vi "TorsionTester.vi"() -> ()   [LabVIEW 2020]
uses:
  C:/Users/elm2733/Box/Rausch Lab/LabView Files/Biaxial Device/MotorPlusLoadCells2 Folder v2016/FUTEK USB DLL.dll
  Box/Rausch Lab/LabView Files/Biaxial Device/MotorPlusLoadCells2 Folder v2016/FUTEK USB DLL.dll
  aec8d69f-4215-41ae-99f2-a40d43009400.vi
  f842f3ff-62f7-4fe2-ab09-e212065798b6.vi
  79f05c57-3d67-4982-bbb2-fea1714bb2cf.vi
  <vilib>/Array/Sort 2D Array - Pop Stack.vi
  <vilib>/Array/Sort 2D Array - Push Stack.vi
  aec8d69f-4215-41ae-99f2-a40d43009400.vi/269d4b3b-47f5-49e3-8884-44851e4dd9d5.vi
  aec8d69f-4215-41ae-99f2-a40d43009400.vi/6d99389c-673d-4efb-bf33-19b32bcf4cf8.vi
  f842f3ff-62f7-4fe2-ab09-e212065798b6.vi/269d4b3b-47f5-49e3-8884-44851e4dd9d5.vi
  f842f3ff-62f7-4fe2-ab09-e212065798b6.vi/6d99389c-673d-4efb-bf33-19b32bcf4cf8.vi
  79f05c57-3d67-4982-bbb2-fea1714bb2cf.vi/269d4b3b-47f5-49e3-8884-44851e4dd9d5.vi
  79f05c57-3d67-4982-bbb2-fea1714bb2cf.vi/6d99389c-673d-4efb-bf33-19b32bcf4cf8.vi
  <vilib>/Utility/file.llb/Write Delimited Spreadsheet (string).vi
  <vilib>/Utility/file.llb/Write Delimited Spreadsheet (DBL).vi
  <vilib>/express/express arith-compare/Formula/XNode/ExpressFormulaBlockNode.xnode
  Box/Rausch Lab/LabView Files/Biaxial Device/MotorPlusLoadCells2 Folder v2016/Zaber A Series/Zaber A Series.lvlib
panel:
  in  "Uniaxial Compression Test":bool
  in  "Uniaxial Tensile Test":bool
  in  "Compression (mm)":dbl format="%#_13g"
  in  "1 Step Test Button":bool
  in  "Cyclic Test Button":bool
  out "error out":errorcluster
  in  "Home Z Motor":bool
  in  "Cycles":i32
  in  "Step Size (mm)":dbl format="%#_13g"
  in  "Down":bool=TRUE
  in  "Up":bool=TRUE
  out "Z Motor Initialized":bool=TRUE
  in  "Motor Speed (mm/s)":dbl format="%#_13g"
  out "Force Sensor (lbs)":dbl format="%#_13g"
  in  "Zero Force Sensor":bool
  in  "Exit Loop":bool=TRUE
  out "Uniaxial Test":bool=TRUE
  out "Uniaxial Cycles":dbl format="%#_13g"
  out "Force/Time":dbl[](graph)
  out "Get_Decimal Point 3":string
  out "Get_Fullscale_Load 3":string
  out "Get_Fullscale_Value 3":string
  out "Get_Offset_Load 3":string
  out "Get_Offset_Value 3":string
  out "1/x 3":dbl format="%#_13g"
  out "Displacement/Time":sgl[](graph)
  in  "Displacement (mm)":dbl format="%#_13g"
  in  "Z Motor":refnum<k7>(container)
  out "Saved Position":dbl[](array[numeric])
  out "Position (Degrees)":dbl=6.0
  in  "Jog Graphs":bool
  out "On/Off":bool
  in  "Record Data":bool
  in  "Save Folder Path":path=path "C:/Users/kv8453/Desktop/LabVIEW_project_PB_tester/Output"
  in  "Sample Name":string="trial"
  out "1/x 2":dbl
  in  "Sampling Rate (Hz)":dbl
  out "Torque Sensor (in-oz)":dbl
  in  "Zero Torque Sensor":bool
  in  "Save Button":bool
  out "Torque/Time":dbl[](graph)
  out "Get_Decimal Point 2":string
  out "Get_Fullscale_Load 2":string
  out "Get_Fullscale_Value 2":string
  out "Get_Offset_Load 2":string
  out "Get_Offset_Value 2":string
  out "1/x":dbl
  in  "Angle (Degrees)":dbl=6.0
  in  "Move Distance (Deg)":dbl=6.0
  in  "Jog Size (Degrees)":dbl=6.0
  out "Angle/Time":dbl[](graph)
  in  "Home Button":bool
  in  "CW Button":bool
  in  "CCW Button":bool
  in  "Speed (Deg/s)":dbl=6.0
  out "Current Cycle":dbl
  in  "Cycles":i32=3
  in  "Quit":bool
  in  "VISA resource name":refnum<visa-resource-name>="COM4"
  # "Torsional Shear Tester                  X                       Uniaxial Tensile Tester"
  # "Rotation Stage = Yellow"
  # "Z Stage = Blue"
  # "Manuel Rausch"
  # "Ethan Maddin"
  # "Jog"
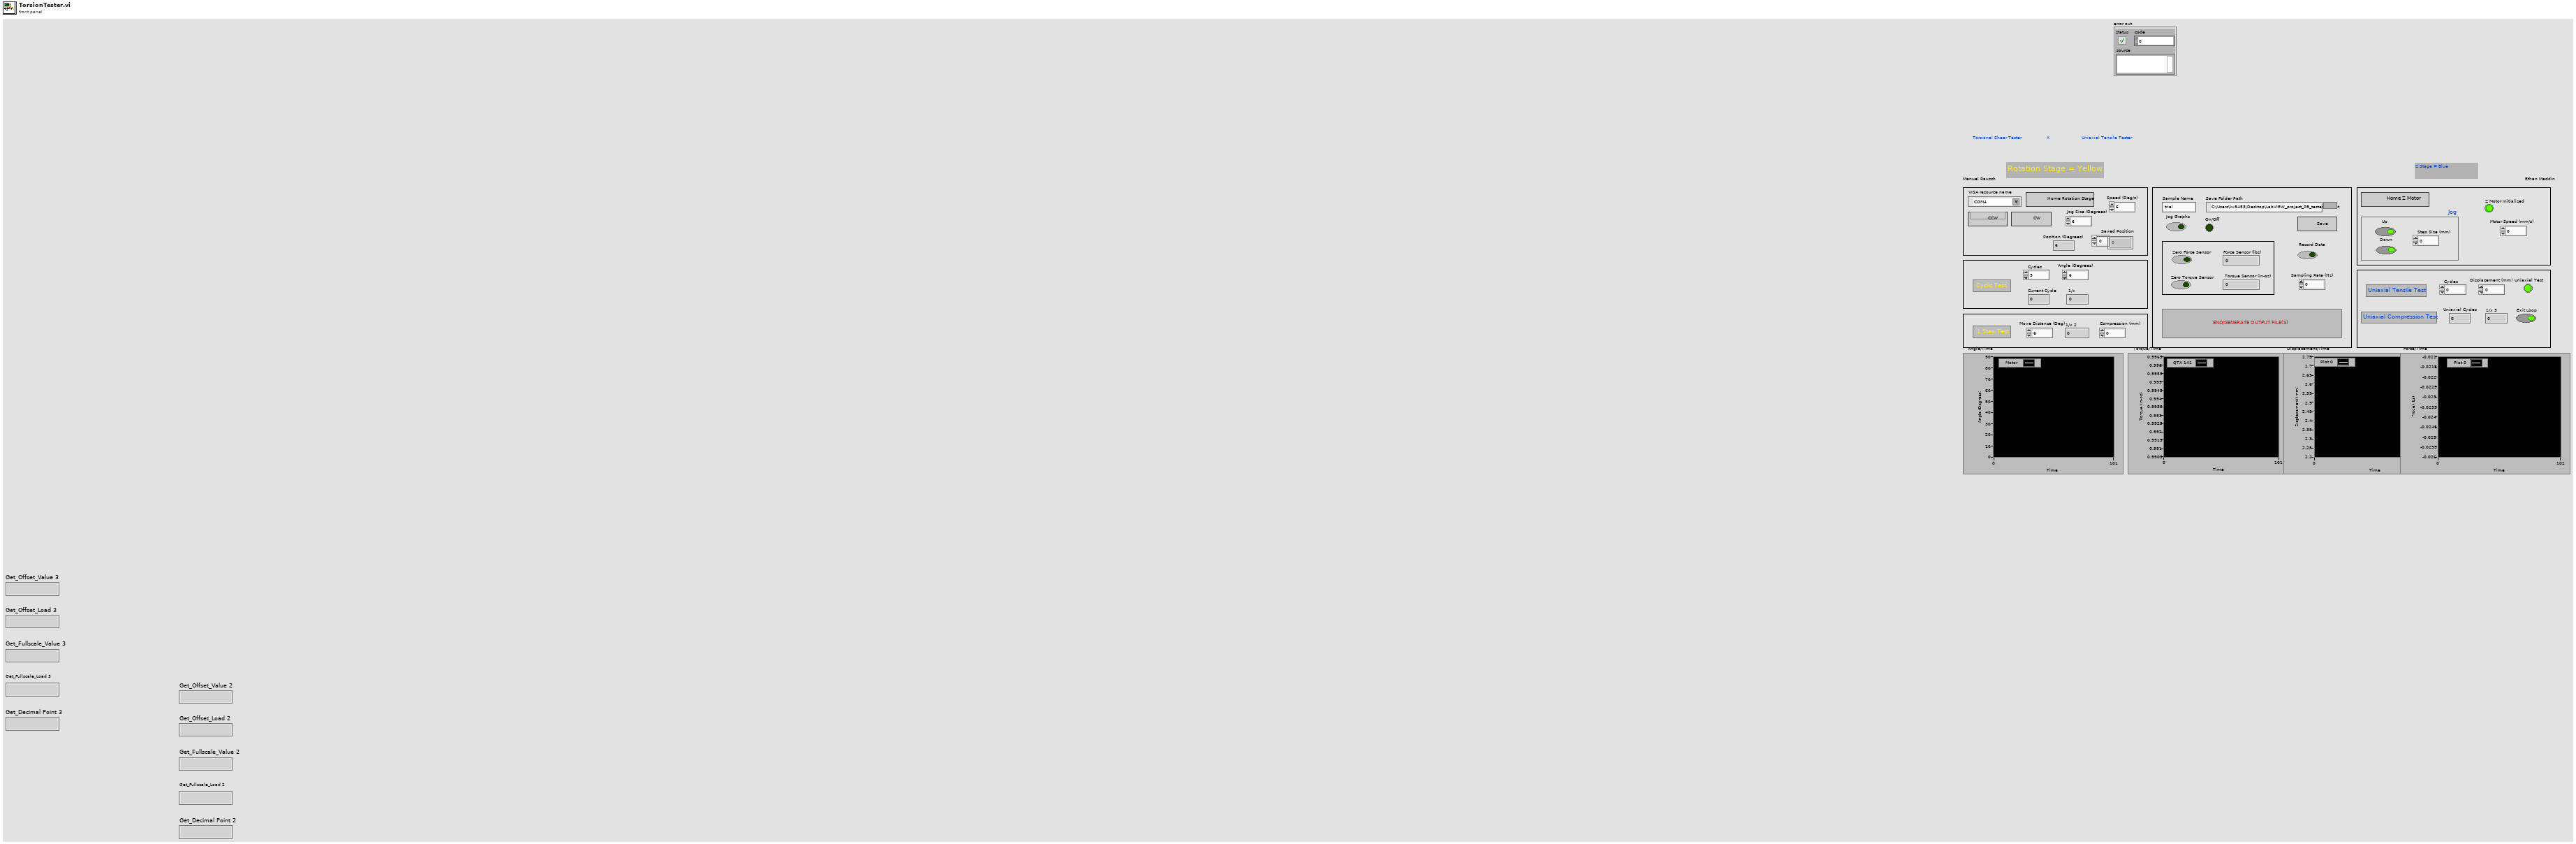
[diagram p1: front panel]
types:
  T1 = enum8{"Enabled", "Disabled", "Disabled and Grayed Out"}
  T2 = cluster{i32, i32, i32, i32, "new reference":refnum<k24>, "DeviceHandle":string, dbl}
  T3 = cluster{"new reference":refnum<k24>, "DeviceHandle":string}
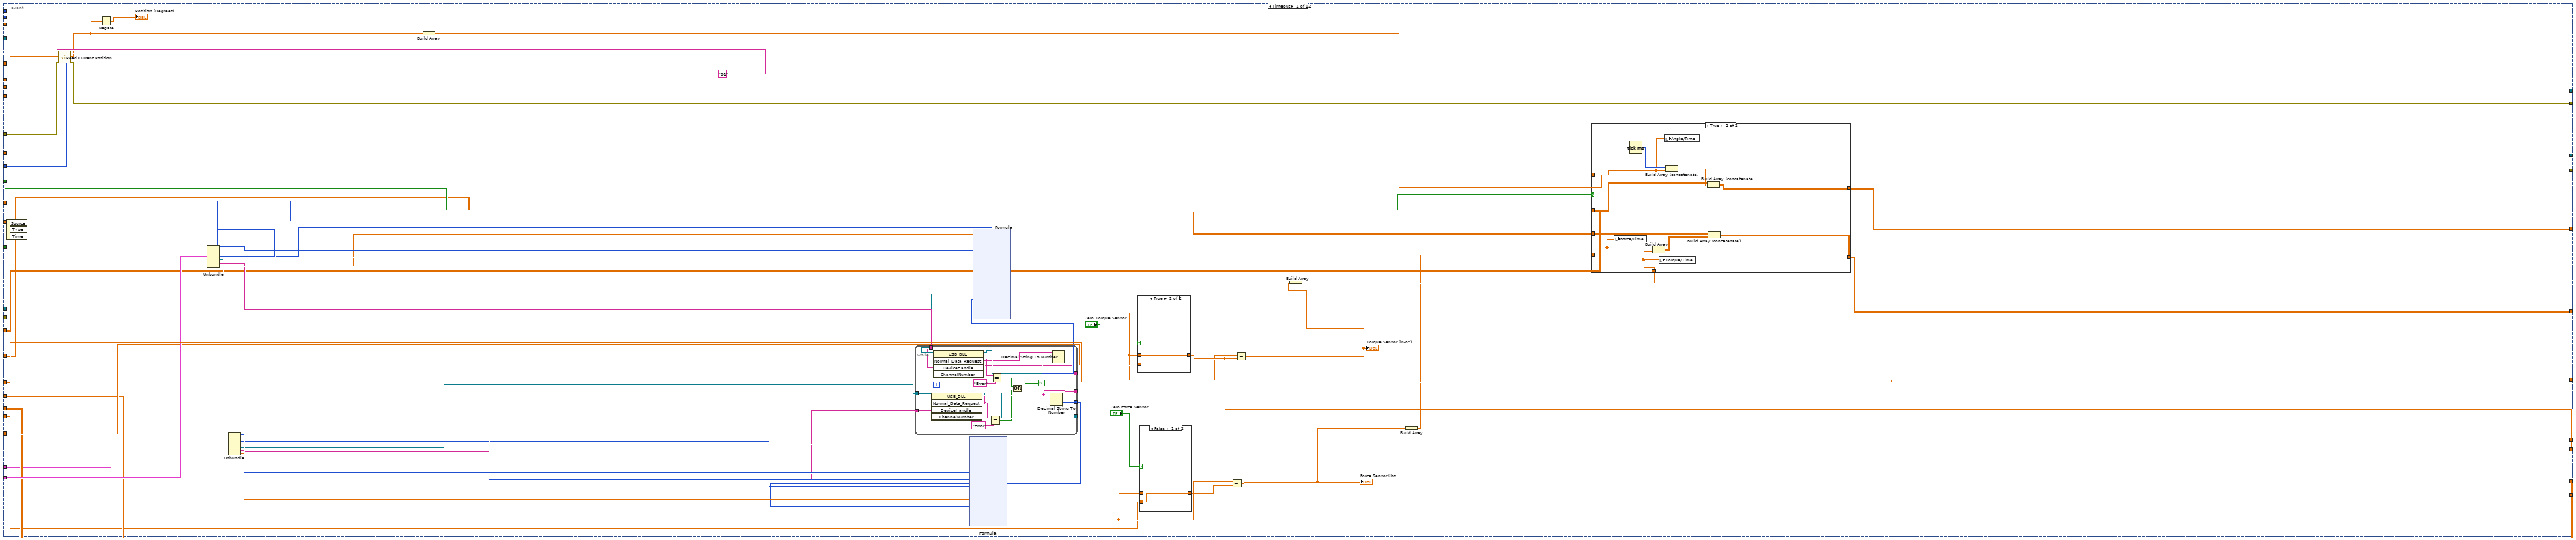
[diagram p2: hidden frame]
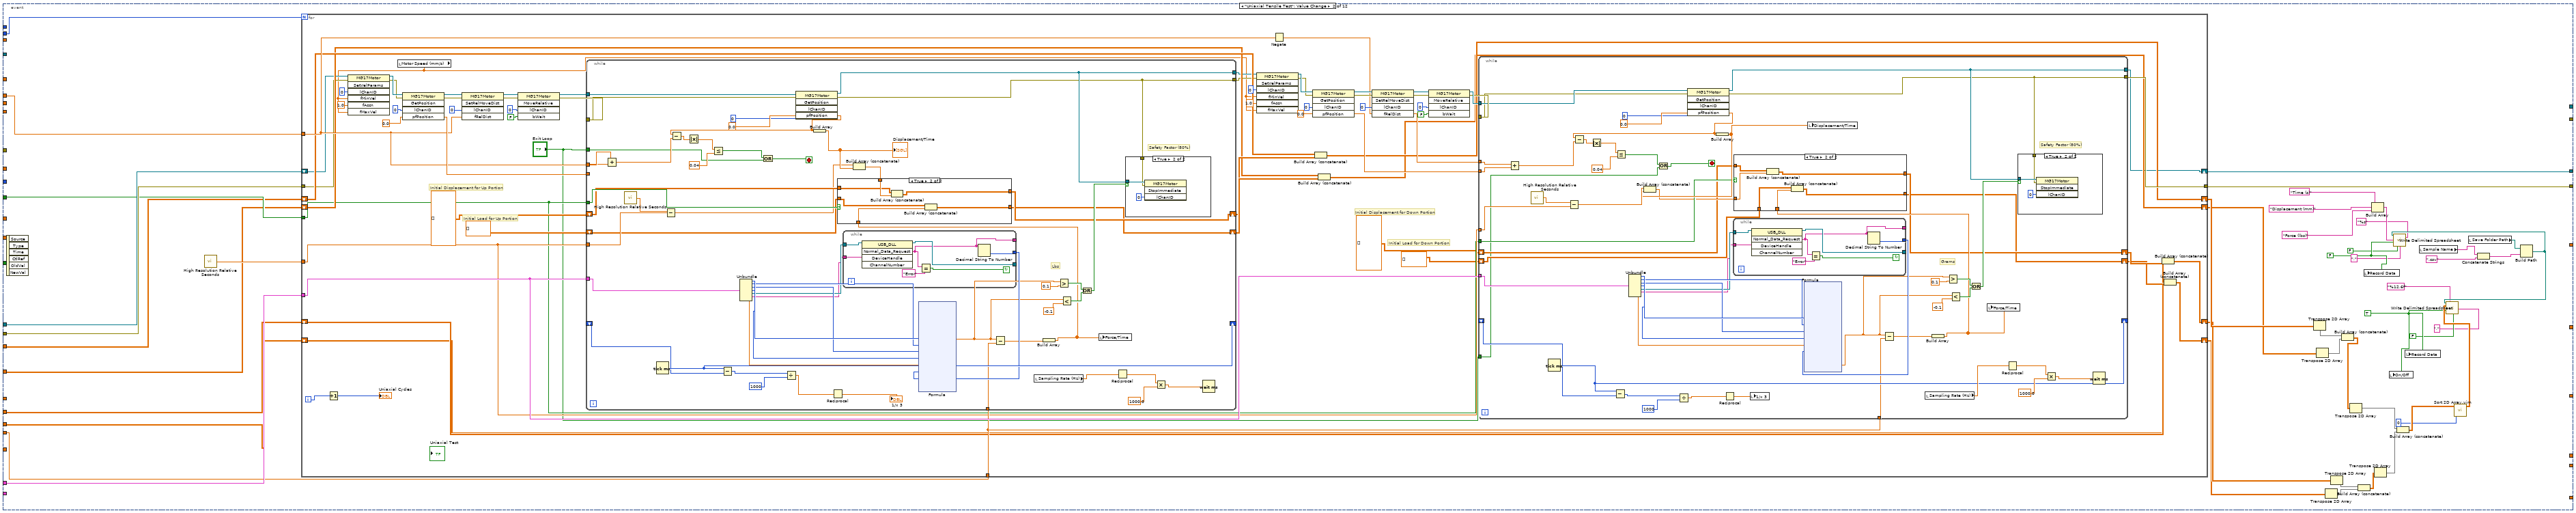
[diagram p6: hidden frame]
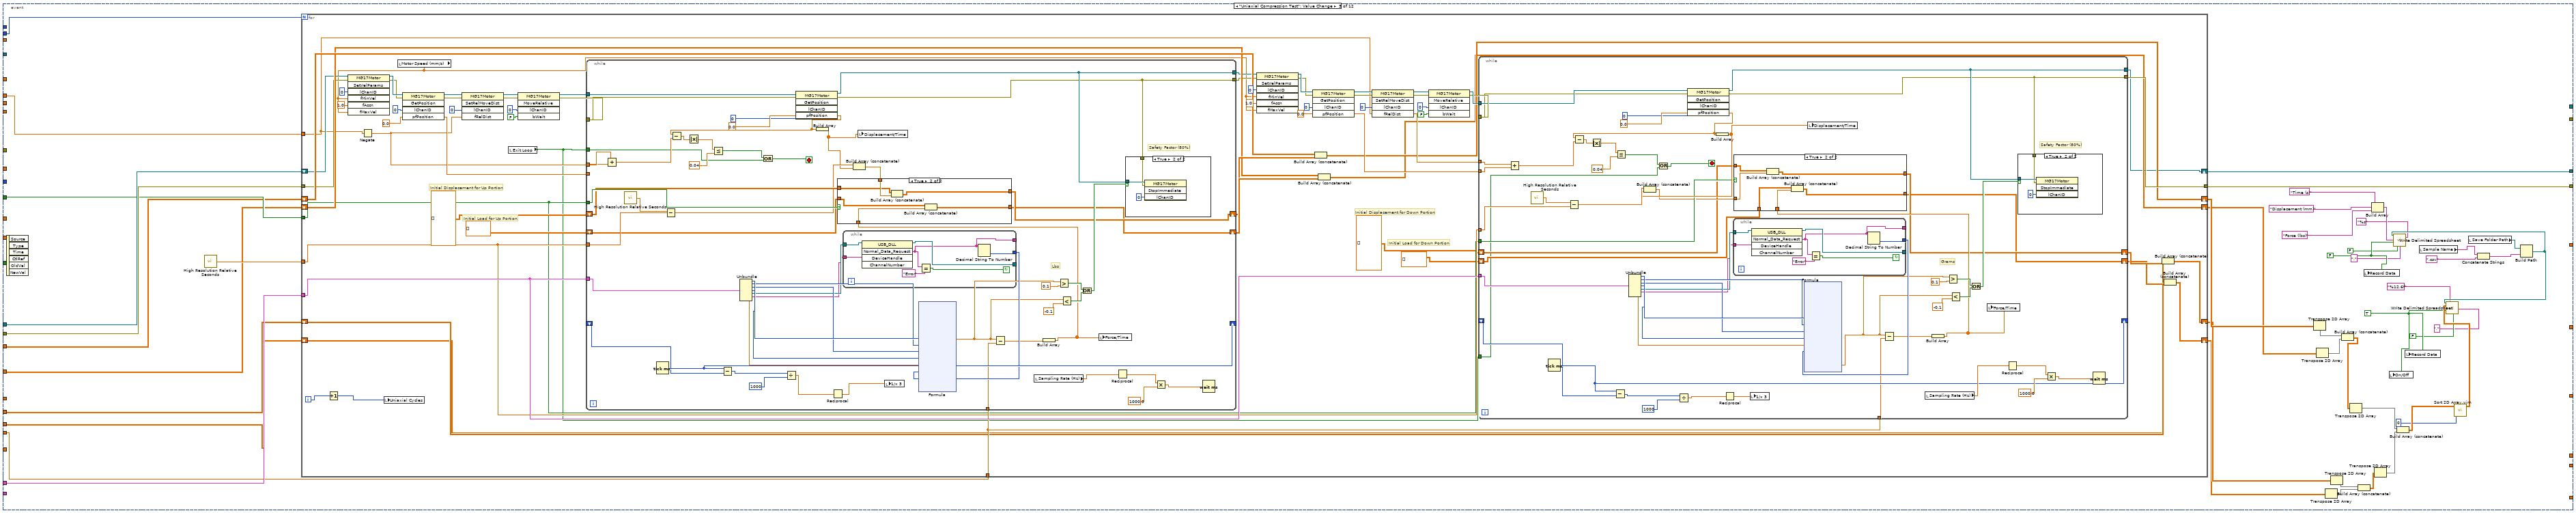
[diagram p11: hidden frame]
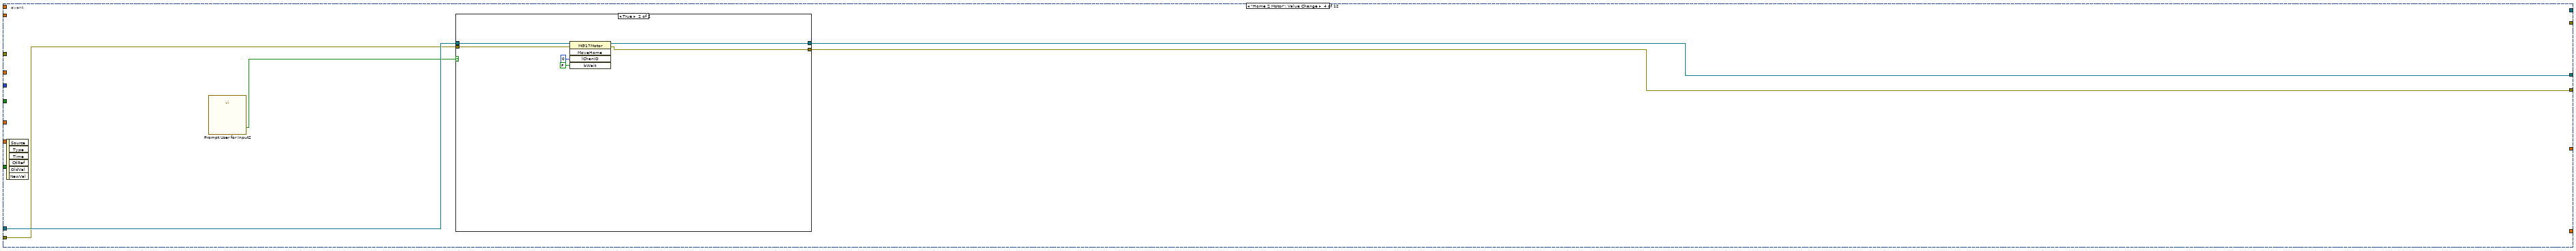
[diagram p16: hidden frame]
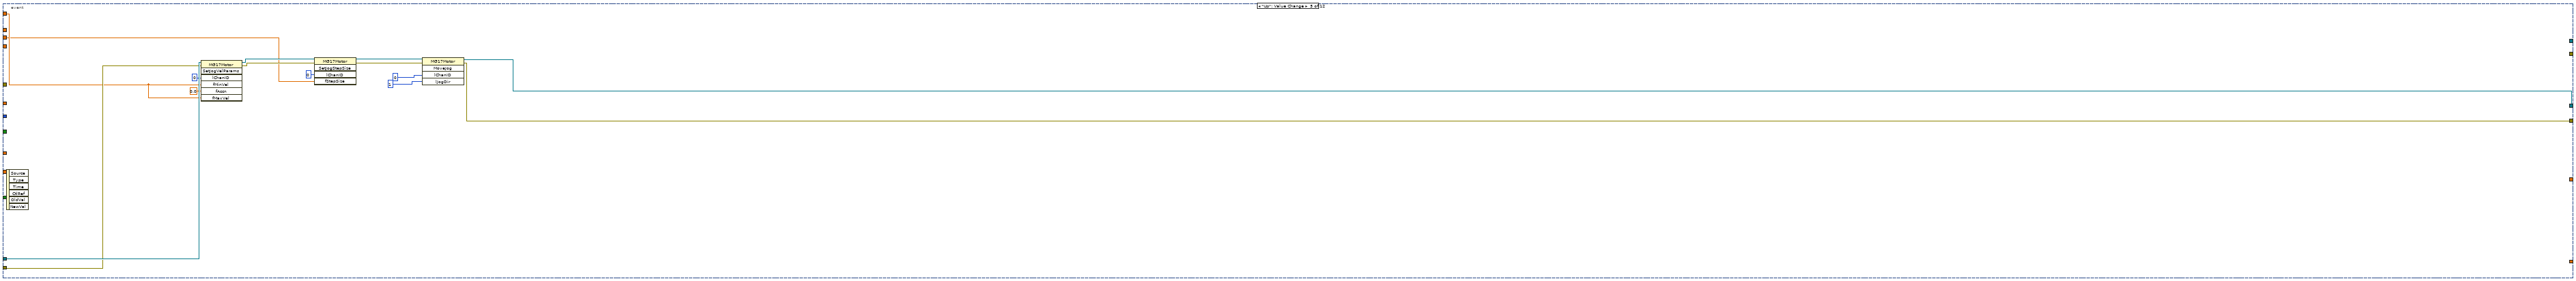
[diagram p18: hidden frame]
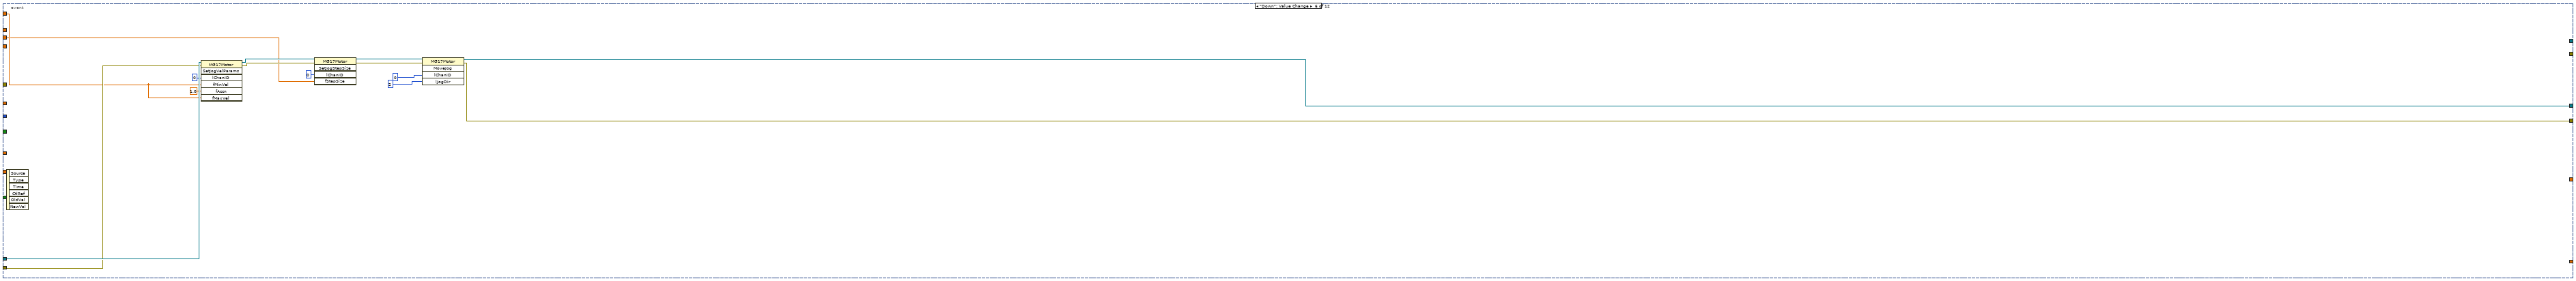
[diagram p19: hidden frame]
diagram:
  # "Sensor Data 2"
  # "Motor Exporting Data 2"
  # "Sensor Data 1"
  # "Motor Exporting Data 1"
  n1 = flat-sequence {
    tunnel: [w71] -> w22
    tunnel: [w70] -> w19
    tunnel: [dbl[] []] -> w21
    tunnel: [w51] -> w16
    tunnel: [w28] -> w7
    tunnel: [w27] -> w6
    tunnel: [w29] -> w4
    frame #0 {
      n2 = invoke on="Down" class="Bool (strict)" method="Reinit To Default"() -> ()  [unwired: 3 in, 3 out]
      n3 = invoke on="On/Off" class="Bool (strict)" method="Reinit To Default"() -> ()  [unwired: 3 in, 3 out]
      n4 = invoke on="Up" class="Bool (strict)" method="Reinit To Default"() -> ()  [unwired: 3 in, 3 out]
      n5 = invoke on="Uniaxial Test" class="Bool (strict)" method="Reinit To Default"() -> ()  [unwired: 3 in, 3 out]
      n6 = invoke on="Z Motor Initialized" class="Bool (strict)" method="Reinit To Default"() -> ()  [unwired: 3 in, 3 out]
    }
    frame #1 {
      n7 = constructor class="USB_DLL"() -> (reference out=w59:refnum<k24>)  [unwired: 3 in, 2 out]
      n8 = constructor class="USB_DLL"() -> (reference out=w37:refnum<k24>)  [unwired: 3 in, 2 out]
      n9 = invoke class="USB_DLL" method="Open_Device_Connection"(reference=w59, "SerialNumber"="1016700" ("Enter Serial Number")) -> (reference out=w61:refnum<k24>)  [unwired: 2 in, 3 out]
      n10 = invoke class="USB_DLL" method="Open_Device_Connection"(reference=w37, "SerialNumber"="905894" ("Enter Serial Number")) -> (reference out=w39:refnum<k24>)  [unwired: 2 in, 3 out]
      n11 = property class="USB_DLL"(reference=w61) -> (reference out=w67:refnum<k24>, "DeviceHandle"=w52:string)  [unwired: 1 in, 1 out]
      n12 = property class="USB_DLL"(reference=w39) -> (reference out=w45:refnum<k24>, "DeviceHandle"=w30:string)  [unwired: 1 in, 1 out]
      n13 = while {
        tunnel: w67 -> [w143]
        tunnel: w52 -> [w142]
        tunnel: [w138] -> w58
        tunnel: [w137] -> w65
        stop <- w139 continue-if-true
        # "Get_Offset_Value is used to read the ADC value stored in the USB device for a zero mV/V load."
        n14 = invoke class="USB_DLL" method="Get_Offset_Value"(reference=w143, "DeviceHandle"=w142) -> (reference out=w137:refnum<k24>, "Get_Offset_Value"=w141:string)  [unwired: 3 in, 3 out]
        "Get_Offset_Value 2" <- w141
        n15 = Equal?(x=w141, y="Error") -> (x = y?=w139:bool)
        n16 = Decimal String To Number(string=w141) -> (number=w138:i32)  [unwired: 2 in, 1 out]
      }
      n17 = while {
        tunnel: w45 -> [w108]
        tunnel: w30 -> [w107]
        tunnel: [w103] -> w36
        tunnel: [w102] -> w43
        stop <- w104 continue-if-true
        # "Get_Offset_Value is used to read the ADC value stored in the USB device for a zero mV/V load."
        n18 = invoke class="USB_DLL" method="Get_Offset_Value"(reference=w108, "DeviceHandle"=w107) -> (reference out=w102:refnum<k24>, "Get_Offset_Value"=w106:string)  [unwired: 3 in, 3 out]
        "Get_Offset_Value 3" <- w106
        n19 = Equal?(x=w106, y="Error") -> (x = y?=w104:bool)
        n20 = Decimal String To Number(string=w106) -> (number=w103:i32)  [unwired: 2 in, 1 out]
      }
      n21 = while {
        tunnel: [w133] -> w57
        tunnel: [w132] -> w64
        tunnel: w65 -> [w131]
        tunnel: w52 -> [w130]
        stop <- w134 continue-if-true
        # "Get_Offset_Load is used to read the capacity of the zero load value stored in the USB device."
        n22 = invoke class="USB_DLL" method="Get_Offset_Load"(reference=w131, "DeviceHandle"=w130) -> (reference out=w132:refnum<k24>, "Get_Offset_Load"=w136:string)  [unwired: 3 in, 3 out]
        "Get_Offset_Load 2" <- w136
        n23 = Equal?(x=w136, y="Error") -> (x = y?=w134:bool)
        n24 = Decimal String To Number(string=w136) -> (number=w133:i32)  [unwired: 2 in, 1 out]
      }
      n25 = while {
        tunnel: [w98] -> w35
        tunnel: [w97] -> w42
        tunnel: w43 -> [w96]
        tunnel: w30 -> [w95]
        stop <- w99 continue-if-true
        # "Get_Offset_Load is used to read the capacity of the zero load value stored in the USB device."
        n26 = invoke class="USB_DLL" method="Get_Offset_Load"(reference=w96, "DeviceHandle"=w95) -> (reference out=w97:refnum<k24>, "Get_Offset_Load"=w101:string)  [unwired: 3 in, 3 out]
        "Get_Offset_Load 3" <- w101
        n27 = Equal?(x=w101, y="Error") -> (x = y?=w99:bool)
        n28 = Decimal String To Number(string=w101) -> (number=w98:i32)  [unwired: 2 in, 1 out]
      }
      n29 = while {
        tunnel: [w126] -> w56
        tunnel: [w125] -> w63
        tunnel: w64 -> [w124]
        tunnel: w52 -> [w123]
        stop <- w127 continue-if-true
        # "Get_Fullscale_Value is used to read the ADC value stored in the USB device for a full load."
        n30 = invoke class="USB_DLL" method="Get_Fullscale_Value"(reference=w124, "DeviceHandle"=w123) -> (reference out=w125:refnum<k24>, "Get_Fullscale_Value"=w129:string)  [unwired: 3 in, 3 out]
        "Get_Fullscale_Value 2" <- w129
        n31 = Equal?(x=w129, y="Error") -> (x = y?=w127:bool)
        n32 = Decimal String To Number(string=w129) -> (number=w126:i32)  [unwired: 2 in, 1 out]
      }
      n33 = while {
        tunnel: [w91] -> w34
        tunnel: [w90] -> w41
        tunnel: w42 -> [w89]
        tunnel: w30 -> [w88]
        stop <- w92 continue-if-true
        # "Get_Fullscale_Value is used to read the ADC value stored in the USB device for a full load."
        n34 = invoke class="USB_DLL" method="Get_Fullscale_Value"(reference=w89, "DeviceHandle"=w88) -> (reference out=w90:refnum<k24>, "Get_Fullscale_Value"=w94:string)  [unwired: 3 in, 3 out]
        "Get_Fullscale_Value 3" <- w94
        n35 = Equal?(x=w94, y="Error") -> (x = y?=w92:bool)
        n36 = Decimal String To Number(string=w94) -> (number=w91:i32)  [unwired: 2 in, 1 out]
      }
      n37 = property class="MG17Motor"(reference="Z Motor", error in=errorcluster {"status"=FALSE, "code"=0, "source"=""}, "HWSerialNum"=27262533 ("HWSerialNum 3")) -> (reference out=w24:refnum<k7>, error out=w23:errorcluster)
      n38 = invoke class="MG17Motor" method="StartCtrl"(reference=w24, error in=w23) -> (reference out=w46:refnum<k7>, error out=w47:errorcluster)  [unwired: 1 in, 1 out]
      n39 = while {
        tunnel: [w119] -> w55
        tunnel: [w118] -> w62
        tunnel: w63 -> [w117]
        tunnel: w52 -> [w116]
        stop <- w120 continue-if-true
        # "Get_Fullsacle_Load is used to read the capacity of the full load value stored in the USB device."
        n40 = invoke class="USB_DLL" method="Get_Fullscale_Load"(reference=w117, "DeviceHandle"=w116) -> (reference out=w118:refnum<k24>, "Get_Fullscale_Load"=w122:string)  [unwired: 3 in, 3 out]
        "Get_Fullscale_Load 2" <- w122
        n41 = Equal?(x=w122, y="Error") -> (x = y?=w120:bool)
        n42 = Decimal String To Number(string=w122) -> (number=w119:i32)  [unwired: 2 in, 1 out]
      }
      n43 = while {
        tunnel: [w84] -> w33
        tunnel: [w83] -> w40
        tunnel: w41 -> [w82]
        tunnel: w30 -> [w81]
        stop <- w85 continue-if-true
        # "Get_Fullsacle_Load is used to read the capacity of the full load value stored in the USB device."
        n44 = invoke class="USB_DLL" method="Get_Fullscale_Load"(reference=w82, "DeviceHandle"=w81) -> (reference out=w83:refnum<k24>, "Get_Fullscale_Load"=w87:string)  [unwired: 3 in, 3 out]
        "Get_Fullscale_Load 3" <- w87
        n45 = Equal?(x=w87, y="Error") -> (x = y?=w85:bool)
        n46 = Decimal String To Number(string=w87) -> (number=w84:i32)  [unwired: 2 in, 1 out]
      }
      n47 = invoke class="MG17Motor" method="GetHWCommsOK"(reference=w46, error in=w47, "pbCommsOK"=FALSE) -> (reference out=w28:refnum<k7>, error out=w27:errorcluster, "pbCommsOK"=→"Z Motor Initialized":bool)  [unwired: 1 in, 1 out]
      n48 = call "Initialize.vi"("error in (no error)"=errorcluster {"status"=FALSE, "code"=0, "source"=""}, "VISA resource name"="VISA resource name") -> ("error out"=w70:errorcluster, "VISA resource name out"=w71:refnum<visa-resource-name>)  [unwired: 8 in]
      n49 = while {
        tunnel: [w112] -> w66
        tunnel: [w111] -> w53
        tunnel: w62 -> [w110]
        tunnel: w52 -> [w109]
        stop <- w113 continue-if-true
        # "Get_Decimal_Point is used to read the position of the decimal point stored in the USB device.  The decimal point is then turned into a negative power of 10."
        n50 = invoke class="USB_DLL" method="Get_Decimal_Point"(reference=w110, "DeviceHandle"=w109) -> (reference out=w111:refnum<k24>, "Get_Decimal_Point"=w115:string)  [unwired: 3 in, 3 out]
        "Get_Decimal Point 2" <- w115
        n51 = Equal?(x=w115, y="Error") -> (x = y?=w113:bool)
        n52 = Decimal String To Number(string=w115) -> (number=w112:i32)  [unwired: 2 in, 1 out]
      }
      n53 = while {
        tunnel: [w77] -> w44
        tunnel: [w76] -> w31
        tunnel: w40 -> [w75]
        tunnel: w30 -> [w74]
        stop <- w78 continue-if-true
        # "Get_Decimal_Point is used to read the position of the decimal point stored in the USB device.  The decimal point is then turned into a negative power of 10."
        n54 = invoke class="USB_DLL" method="Get_Decimal_Point"(reference=w75, "DeviceHandle"=w74) -> (reference out=w76:refnum<k24>, "Get_Decimal_Point"=w80:string)  [unwired: 3 in, 3 out]
        "Get_Decimal Point 3" <- w80
        n55 = Equal?(x=w80, y="Error") -> (x = y?=w78:bool)
        n56 = Decimal String To Number(string=w80) -> (number=w77:i32)  [unwired: 2 in, 1 out]
      }
      n57 = Power Of 10(x=w66) -> (10^x=w54:dbl)
      n58 = Power Of 10(x=w44) -> (10^x=w32:dbl)
      n59 = property on="Home Button" class="Bool"("DisabledEnum"=T1."Enabled" ("Disabled")) -> ()  [unwired: 2 in, 2 out]
      n60 = Bundle(w58, w57, w56, w55, "new reference"=w53, "DeviceHandle"=w52, w54) -> (w51:T2)  [unwired: 1 in]
      n61 = Bundle(w36, w35, w34, w33, "new reference"=w31, "DeviceHandle"=w30, w32) -> (w29:T2)  [unwired: 1 in]
    }
  }
  n62 = while {
    tunnel: w22 -> [w187]
    tunnel: [w184] -> w20
    shift-right: [w183] -> w13
    shift-left: w19 -> [w182]
    shift-right: [w164] -> w8
    shift-left: w21 -> [w181]
    shift-right: [w175] -> _
    shift-left: 0.0 -> [w177]
    shift-right: [w174] -> _
    shift-left: 0.0 -> [w176]
    tunnel: w16 -> [w173]
    tunnel: [w169] -> w15
    tunnel: [w168] -> w14
    tunnel: dbl[][] [] ("Array") -> [w163]
    tunnel: dbl[][] [] ("Array") -> [w161]
    tunnel: dbl[][] [] ("Array") -> [w160]
    tunnel: dbl[][] [] ("Array") -> [w159]
    tunnel: w6 -> [w156]
    tunnel: [w155] -> w5
    tunnel: w4 -> [w154]
    tunnel: [w150] -> w3
    tunnel: [w149] -> w2
    tunnel: w7 -> [w157]
    tunnel: [w147] -> w1
    stop <- "Quit" stop-if-true
    w185 = u16 4 items=["microsteps", "microns", "millimeters", "inches", "degrees"] ("Units (0: microsteps)")
    # "Uniaxial"
    # "Torsional Shear"
    n63 = Unbundle By Name(w173) -> ("new reference"=w172:refnum<k24>, "DeviceHandle"=w171:string)
    n64 = Unbundle By Name(w154) -> ("new reference"=w153:refnum<k24>, "DeviceHandle"=w152:string)
    n65 = event shown="[6] \"1 Step Test Button\": Value Change" {
      selector: _ -> [_ _ _ _ _ _ _ _ _ _ _ _]
      dyn-events: _ -> [_ _ _ _ _ _ _ _ _ _ _ _]
      timeout: u32 10 ("millisecond timer value") -> [_ _ _ _ _ _ _ _ _ _ _ _]
      tunnel: "Cycles" -> [_ _ _ _ _ _ _ w1249 _ _ _ _]
      tunnel: w187 -> [w234 _ _ _ _ _ w974 w1248 w1593 w1666 w1727 w1752]
      tunnel: 0.000234375 -> [w237 _ _ _ _ _ w972 w1247 w1596 w1667 _ w1754]
      tunnel: w185 -> [w236 _ _ _ _ _ w982 w1246 w1595 w1668 _ w1753]
      tunnel: [w232 _ _ _ _ _ w979 w1245 w1581 w1652 w1725 w1749] -> w184
      tunnel: [w231 _ _ _ _ _ w978 w1244 w1580 w1651 w1724 w1748] -> w183
      tunnel: w182 -> [w235 _ _ _ _ _ w973 w1243 w1592 w1665 w1728 w1751]
      tunnel: "Jog Size (Degrees)" -> [_ _ _ _ _ _ _ _ w1597 w1670 _ _]
      tunnel: w181 -> [w230 _ _ _ _ _ w960 w1242 w1590 w1662 w1735 _]
      tunnel: [w230 _ _ _ _ _ w959 w1242 w1590 w1662 w1735 w1745] -> w164
      tunnel: "Move Distance (Deg)" -> [_ _ _ _ _ _ w962 _ _ _ _ _]
      tunnel: "Angle (Degrees)" -> [_ _ _ _ _ _ _ w1241 _ _ _ _]
      tunnel: w177 -> [w192 w345 w636 _ _ _ w977 w1238 w1589 w1661 w1734 w1747]
      tunnel: w176 -> [w221 _ _ _ _ _ w976 w1237 w1588 w1660 w1733 w1746]
      tunnel: [_ _ _ _ _ _ w977 w1238 w1589 w1661 w1734 w1747] -> w175
      tunnel: [w220 _ _ _ _ _ w976 w1237 w1588 w1660 w1733 w1746] -> w174
      tunnel: w173 -> [w229 _ _ _ _ _ w975 w1239 w1584 w1655 _ _]
      tunnel: "Record Data" -> [_ w344 w635 _ _ _ w971 w1236 _ _ _ _]
      tunnel: [w216 _ _ _ _ _ _ _ w1587 w1659 w1732 _] -> _
      tunnel: w163 -> [w217 w342 w633 _ _ _ w968 w1235 w1587 w1659 w1732 _]
      tunnel: "Jog Graphs" -> [w215 _ _ _ _ _ _ _ _ _ _ _]
      tunnel: w161 -> [w213 w341 w632 _ _ _ w965 w1234 _ w1658 w1731 _]
      tunnel: [w212 _ _ _ _ _ _ _ _ w1658 w1731 _] -> _
      tunnel: w160 -> [w210 w340 w631 _ _ _ w964 w1233 w1586 w1657 w1730 _]
      tunnel: w159 -> [w209 w339 w630 _ _ _ w963 w1232 w1585 w1656 w1729 _]
      tunnel: [w210 _ _ _ _ _ w964 _ w1586 w1657 w1730 _] -> _
      tunnel: [w209 _ _ _ _ _ w963 _ w1585 w1656 w1729 _] -> _
      tunnel: "Displacement (mm)" -> [_ w348 w639 _ _ _ _ _ _ _ _ _]
      tunnel: w157 -> [_ w350 w641 w891 w914 w929 w954 _ _ _ _ _]
      tunnel: w156 -> [_ w349 w640 w890 w913 w928 w953 _ _ _ _ _]
      tunnel: [_ w306 w597 w888 w901 w916 w945 _ _ _ _ _] -> w147
      tunnel: [_ w347 w638 w887 w900 w915 w944 _ _ _ _ _] -> w155
      tunnel: w154 -> [w205 w346 w637 _ _ _ w956 w1198 _ _ _ _]
      tunnel: "Motor Speed (mm/s)" -> [_ _ _ _ w910 w925 w952 _ _ _ _ _]
      tunnel: "Step Size (mm)" -> [_ _ _ _ w906 w921 _ _ _ _ _ _]
      tunnel: "Cycles" -> [_ w305 w596 _ _ _ _ _ _ _ _ _]
      tunnel: "Compression (mm)" -> [_ _ _ _ _ _ w955 _ _ _ _ _]
      event Timeout {
        n66 = event-data() -> ()  [unwired: 1 in, 3 out]
        n67 = call "Read Current Position.vi"("Units (0: microsteps)"=w236, "error in (no error)"=w235, "Device and Axis"="01", "Microstep Size (0)"=w237, "VISA resource name"=w234) -> ("error out"=w231:errorcluster, "Position"=w208:dbl, "VISA resource name out"=w232:refnum<visa-resource-name>)  [unwired: 4 in]
        n68 = Negate(x=w208) -> (-x=→"Position (Degrees)":dbl)
        n69 = Unbundle(w229) -> (w228:i32, w227:i32, w226:i32, w225:i32, "new reference"=w222:refnum<k24>, "DeviceHandle"=w223:string, w224:dbl)
        n70 = Unbundle(w205) -> (w203:i32, w202:i32, w201:i32, w200:i32, "new reference"=w198:refnum<k24>, "DeviceHandle"=w197:string, w199:dbl)
        n71 = Build Array(w208) -> (w218:dbl[])
        n72 = while {
          tunnel: [w285] -> w219
          tunnel: w222 -> [w284]
          tunnel: [w283] -> _
          tunnel: w223 -> [w282]
          tunnel: [w281] -> _
          tunnel: w198 -> [w279]
          tunnel: w197 -> [w278]
          tunnel: [w277] -> _
          tunnel: [w276] -> _
          tunnel: [w275] -> w196
          stop <- w272 continue-if-true
          n73 = invoke class="USB_DLL" method="Normal_Data_Request"(reference=w279, "DeviceHandle"=w278) -> (reference out=w277:refnum<k24>, "Normal_Data_Request"=w276:string)  [unwired: 3 in, 3 out]
          n74 = invoke class="USB_DLL" method="Normal_Data_Request"(reference=w284, "DeviceHandle"=w282) -> (reference out=w283:refnum<k24>, "Normal_Data_Request"=w281:string)  [unwired: 3 in, 3 out]
          n75 = Equal?(x=w276, y="Error") -> (x = y?=w273:bool)
          n76 = Equal?(x=w281, y="Error") -> (x = y?=w274:bool)
          n77 = Or(x=w274, y=w273) -> (x .or. y?=w272:bool)
          n78 = Decimal String To Number(string=w276) -> (number=w275:i32)  [unwired: 2 in, 1 out]
          n79 = Decimal String To Number(string=w281) -> (number=w285:i32)  [unwired: 2 in, 1 out]
        }
        n80 = xnode "Formula"("Get_Offset_Value"=w203, "Get_Offset_Load"=w202, "Get_Fullscale_Value"=w201, "Get_Fullscale_Load"=w200, "Get_Decimal_Point"=w199, "Normal_Data_Request"=w196) -> ("Result"=w194:dbl)  [unwired: 1 in, 1 out]
        n81 = xnode "Formula"("Get_Offset_Value"=w228, "Get_Offset_Load"=w227, "Get_Fullscale_Value"=w226, "Get_Fullscale_Load"=w225, "Get_Decimal_Point"=w224, "Normal_Data_Request"=w219) -> ("Result"=w214:dbl)  [unwired: 1 in, 1 out]
        n82 = case shown="True" "Zero Torque Sensor" {
          tunnel: w214 -> [_ w271]
          tunnel: [w270 w271] -> w220
          tunnel: w221 -> [w270 _]
          frame False {
          }
          frame True {
          }
        }
        n83 = case shown="False" "Zero Force Sensor" {
          tunnel: w194 -> [_ w239]
          tunnel: [w238 w239] -> w193
          tunnel: w192 -> [w238 _]
          frame False {
          }
          frame True {
          }
        }
        n84 = Subtract(x=w194, y=w193) -> (x-y=w191:dbl)
        "Force Sensor (lbs)" <- w191
        n85 = Subtract(x=w214, y=w220) -> (x-y=w204:dbl)
        "Torque Sensor (in-oz)" <- w204
        n86 = Build Array(w204) -> (w206:dbl[])
        n87 = Build Array(w191) -> (w190:dbl[])
        n88 = case shown="True" w215 {
          tunnel: w218 -> [_ w265]
          tunnel: w217 -> [w259 w266]
          tunnel: [w259 w268] -> w216
          tunnel: w206 -> [_ w261]
          tunnel: w213 -> [w258 w263]
          tunnel: [w258 w262] -> w212
          tunnel: w190 -> [_ w260]
          frame False {
          }
          frame True {
            n89 = local write "Force/Time"(w260) -> ()
            n90 = Tick Count (ms)() -> (millisecond timer value=w269:u32)
            n91 = Build Array(w260, w261) -> (w264:dbl[][])
            n92 = local write "Torque/Time"(w261) -> ()
            n93 = local write "Angle/Time"(w265) -> ()
            n94 = Build Array (concatenate)(w269, w265) -> (w267:dbl[])
            n95 = Build Array (concatenate)(w266, w267) -> (w268:dbl[][])
            n96 = Build Array (concatenate)(w263, w264) -> (w262:dbl[][])
          }
        }
      }
      event "Uniaxial Tensile Test": Value Change {
        w325 = FALSE
        w319 = TRUE ("append to file? (new file:F)")
        n97 = event-data() -> ()  [unwired: 1 in, 6 out]
        n98 = call <vilib>:"High Resolution Relative Seconds.vi"() -> ("relative seconds"=w343:dbl)
        n99 = for {
          N: w305 -> [_]
          tunnel: w348 -> [w396]
          tunnel: w346 -> [w393]
          tunnel: w345 -> [w388]
          tunnel: w349 -> [w362]
          tunnel: [w387] -> w347
          tunnel: w344 -> [w376]
          tunnel: w343 -> [w385]
          shift-right: [w378] -> w313
          shift-left: w342 -> [w380]
          shift-right: [w377] -> w312
          shift-left: w341 -> [w379]
          shift-right: [w369] -> w311
          shift-left: w340 -> [w371]
          shift-right: [w368] -> w310
          shift-left: w339 -> [w370]
          shift-right: [w352] -> w306
          shift-left: w350 -> [w363]
          i -> [w406]
          # "Initial Displacement for Down Portion"
          # "Initial Load for Down Portion"
          # "Initial Displacement for Up Portion"
          # "Initial Load for Up Portion"
          n100 = Increment(x=w406) -> (x+1=→"Uniaxial Cycles":i32)
          n101 = local read "Motor Speed (mm/s)"() -> (w353:dbl)
          n102 = invoke class="MG17Motor" method="SetVelParams"(reference=w363, error in=w362, "lChanID"=0, "fMinVel"=w353, "fAccn"=sgl 1.0, "fMaxVel"=w353) -> (reference out=w361:refnum<k7>, error out=w360:errorcluster)  [unwired: 1 in, 5 out]
          n103 = invoke class="MG17Motor" method="GetPosition"(reference=w361, error in=w360, "lChanID"=0, "pfPosition"=sgl 0.0) -> (reference out=w410:refnum<k7>, error out=w409:errorcluster, "pfPosition"=w405:sgl)  [unwired: 1 in, 2 out]
          n104 = invoke class="MG17Motor" method="SetRelMoveDist"(reference=w410, error in=w409, "lChanID"=0, "fRelDist"=w396) -> (reference out=w414:refnum<k7>, error out=w413:errorcluster)  [unwired: 1 in, 3 out]
          n105 = invoke class="MG17Motor" method="MoveRelative"(reference=w414, error in=w413, "lChanID"=0, "bWait"=FALSE) -> (reference out=w351:refnum<k7>, error out=w407:errorcluster)  [unwired: 1 in, 3 out]
          n106 = while {
            tunnel: w407 -> [w559]
            shift-right: [w548] -> _
            shift-left: _ -> [w547]
            tunnel: [w523] -> w359
            tunnel: [w521] -> w358
            tunnel: w393 -> [w546]
            tunnel: w388 -> [w537]
            tunnel: w396 -> [w535]
            tunnel: w405 -> [w534]
            tunnel: w385 -> [w519]
            tunnel: w376 -> [w518]
            shift-right: [w511] -> w381
            shift-left: dbl[][] [] ("Array") -> [w517]
            shift-right: [w510] -> w382
            shift-left: dbl[][] [] ("Array") -> [w516]
            tunnel: "Exit Loop" -> [w507]
            tunnel: w351 -> [w506]
            stop <- w508 stop-if-true
            # "Safety Factor (80%)"
            # "Lbs"
            n107 = Add(x=w535, y=w534) -> (x+y=w532:dbl)
            n108 = call <vilib>:"High Resolution Relative Seconds.vi"() -> ("relative seconds"=w520:dbl)
            n109 = Tick Count (ms)() -> (millisecond timer value=w548:u32)
            n110 = Subtract(x=w520, y=w519) -> (x-y=w514:dbl)
            n111 = Subtract(x=w548, y=w547) -> (x-y=w552:u32)
            n112 = Unbundle(w546) -> (w545:i32, w544:i32, w543:i32, w542:i32, "new reference"=w540:refnum<k24>, "DeviceHandle"=w539:string, w541:dbl)
            n113 = Divide(x=w552, y=1000) -> (x/y=w550:dbl)
            n114 = invoke class="MG17Motor" method="GetPosition"(reference=w506, error in=w559, "lChanID"=0, "pfPosition"=sgl 0.0) -> (reference out=w523:refnum<k7>, error out=w521:errorcluster, "pfPosition"=w533:sgl)  [unwired: 1 in, 2 out]
            n115 = Subtract(x=w533, y=w532) -> (x-y=w530:dbl)
            n116 = Absolute Value(x=w530) -> (abs(x)=w529:dbl)
            n117 = Less Or Equal?(x=w529, y=0.04) -> (x <= y?=w509:bool)
            n118 = Or(x=w509, y=w507) -> (x .or. y?=w508:bool)
            n119 = Build Array(w533) -> (w515:sgl[])
            "Displacement/Time" <- w515
            n120 = Reciprocal(x=w550) -> (1/x=→"1/x 3":dbl)
            n121 = while {
              tunnel: [w594] -> _
              tunnel: [w593] -> _
              tunnel: [w592] -> w538
              tunnel: w539 -> [w591]
              tunnel: w540 -> [w590]
              stop <- w589 continue-if-true
              n122 = invoke class="USB_DLL" method="Normal_Data_Request"(reference=w590, "DeviceHandle"=w591) -> (reference out=w594:refnum<k24>, "Normal_Data_Request"=w593:string)  [unwired: 3 in, 3 out]
              n123 = Equal?(x=w593, y="Error") -> (x = y?=w589:bool)
              n124 = Decimal String To Number(string=w593) -> (number=w592:i32)  [unwired: 2 in, 1 out]
            }
            n125 = Build Array (concatenate)(w514, w515) -> (w513:dbl[])
            n126 = xnode "Formula"("Get_Offset_Value"=w545, "Get_Offset_Load"=w544, "Get_Fullscale_Value"=w543, "Get_Fullscale_Load"=w542, "Get_Decimal_Point"=w541, "Normal_Data_Request"=w538) -> ("Result"=w524:dbl)  [unwired: 1 in, 1 out]
            n127 = Subtract(x=w524, y=w537) -> (x-y=w536:dbl)
            n128 = local read "Sampling Rate (Hz)"() -> (w555:dbl)
            n129 = Build Array(w536) -> (w512:dbl[])
            n130 = case shown="True" w518 {
              tunnel: w517 -> [w561 w566]
              tunnel: w516 -> [w560 w565]
              tunnel: w513 -> [_ w567]
              tunnel: w512 -> [_ w564]
              tunnel: [w560 w563] -> w510
              tunnel: [w561 w562] -> w511
              frame False {
              }
              frame True {
                n131 = Build Array (concatenate)(w566, w567) -> (w562:dbl[][])
                n132 = Build Array (concatenate)(w565, w564) -> (w563:dbl[][])
              }
            }
            n133 = Greater?(x=w524, y=0.1) -> (0:w526:bool)
            n134 = Less?(x=w524, y=-0.1) -> (x < y?=w525:bool)
            n135 = Or(x=w526, y=w525) -> (x .or. y?=w522:bool)
            n136 = local write "Force/Time"(w512) -> ()
            n137 = Reciprocal(x=w555) -> (1/x=w554:dbl)
            n138 = case shown="True" w522 {
              tunnel: w523 -> [_ w570]
              tunnel: w521 -> [_ w568]
              frame False {
              }
              frame True {
                n139 = invoke class="MG17Motor" method="StopImmediate"(reference=w570, error in=w568, "lChanID"=0) -> ()  [unwired: 1 in, 4 out]
              }
            }
            n140 = Multiply(x=w554, y=1000.0) -> (x*y=w553:dbl)
            n141 = Wait (ms)(milliseconds to wait=w553) -> ()  [unwired: 1 out]
          }
          n142 = invoke class="MG17Motor" method="SetVelParams"(reference=w359, error in=w358, "lChanID"=0, "fMinVel"=w353, "fAccn"=sgl 1.0, "fMaxVel"=w353) -> (reference out=w357:refnum<k7>, error out=w356:errorcluster)  [unwired: 1 in, 5 out]
          n143 = Negate(x=w396) -> (-x=w395:dbl)
          n144 = invoke class="MG17Motor" method="GetPosition"(reference=w357, error in=w356, "lChanID"=0, "pfPosition"=sgl 0.0) -> (reference out=w399:refnum<k7>, error out=w398:errorcluster, "pfPosition"=w390:sgl)  [unwired: 1 in, 2 out]
          n145 = Build Array (concatenate)(w380, w381) -> (w378:dbl[][])
          n146 = Build Array (concatenate)(w379, w382) -> (w377:dbl[][])
          n147 = invoke class="MG17Motor" method="SetRelMoveDist"(reference=w399, error in=w398, "lChanID"=0, "fRelDist"=w395) -> (reference out=w403:refnum<k7>, error out=w402:errorcluster, "fRelDist"=w389:sgl)  [unwired: 1 in, 2 out]
          n148 = invoke class="MG17Motor" method="MoveRelative"(reference=w403, error in=w402, "lChanID"=0, "bWait"=FALSE) -> (reference out=w392:refnum<k7>, error out=w391:errorcluster)  [unwired: 1 in, 3 out]
          n149 = while {
            tunnel: w392 -> [w469]
            tunnel: w391 -> [w468]
            shift-right: [w458] -> _
            shift-left: _ -> [w457]
            tunnel: [w433] -> w352
            tunnel: [w431] -> w387
            tunnel: w393 -> [w456]
            tunnel: w388 -> [w447]
            tunnel: w389 -> [w445]
            tunnel: w390 -> [w444]
            tunnel: w385 -> [w428]
            tunnel: w376 -> [w425]
            shift-right: [w420] -> w373
            shift-left: dbl[][] [] ("Array") -> [w422]
            shift-right: [w419] -> w372
            shift-left: dbl[][] [] ("Array") -> [w421]
            tunnel: "Exit Loop" -> [w417]
            stop <- w416 stop-if-true
            # "Safety Factor (80%)"
            # "Grams"
            n150 = Add(x=w445, y=w444) -> (x+y=w442:sgl)
            n151 = call <vilib>:"High Resolution Relative Seconds.vi"() -> ("relative seconds"=w429:dbl)
            n152 = Tick Count (ms)() -> (millisecond timer value=w458:u32)
            n153 = Subtract(x=w429, y=w428) -> (x-y=w427:dbl)
            n154 = Subtract(x=w458, y=w457) -> (x-y=w461:u32)
            n155 = Unbundle(w456) -> (w455:i32, w454:i32, w453:i32, w452:i32, "new reference"=w450:refnum<k24>, "DeviceHandle"=w449:string, w451:dbl)
            n156 = Divide(x=w461, y=1000) -> (x/y=w459:dbl)
            n157 = invoke class="MG17Motor" method="GetPosition"(reference=w469, error in=w468, "lChanID"=0, "pfPosition"=sgl 0.0) -> (reference out=w433:refnum<k7>, error out=w431:errorcluster, "pfPosition"=w443:sgl)  [unwired: 1 in, 2 out]
            n158 = Subtract(x=w443, y=w442) -> (x-y=w440:sgl)
            n159 = Absolute Value(x=w440) -> (abs(x)=w439:sgl)
            n160 = Less Or Equal?(x=w439, y=0.04) -> (x <= y?=w418:bool)
            n161 = Or(x=w418, y=w417) -> (x .or. y?=w416:bool)
            n162 = Build Array(w443) -> (w426:sgl[])
            n163 = Build Array (concatenate)(w427, w426) -> (w424:dbl[])
            n164 = Reciprocal(x=w459) -> (1/x=w430:dbl)
            n165 = while {
              tunnel: [w504] -> _
              tunnel: [w503] -> _
              tunnel: [w502] -> w448
              tunnel: w449 -> [w501]
              tunnel: w450 -> [w500]
              stop <- w499 continue-if-true
              n166 = invoke class="USB_DLL" method="Normal_Data_Request"(reference=w500, "DeviceHandle"=w501) -> (reference out=w504:refnum<k24>, "Normal_Data_Request"=w503:string)  [unwired: 3 in, 3 out]
              n167 = Equal?(x=w503, y="Error") -> (x = y?=w499:bool)
              n168 = Decimal String To Number(string=w503) -> (number=w502:i32)  [unwired: 2 in, 1 out]
            }
            n169 = local write "1/x 3"(w430) -> ()
            n170 = xnode "Formula"("Get_Offset_Value"=w455, "Get_Offset_Load"=w454, "Get_Fullscale_Value"=w453, "Get_Fullscale_Load"=w452, "Get_Decimal_Point"=w451, "Normal_Data_Request"=w448) -> ("Result"=w434:dbl)  [unwired: 1 in, 1 out]
            n171 = local write "Displacement/Time"(w426) -> ()
            n172 = Subtract(x=w434, y=w447) -> (x-y=w446:dbl)
            n173 = local read "Sampling Rate (Hz)"() -> (w464:dbl)
            n174 = Build Array(w446) -> (w423:dbl[])
            n175 = case shown="True" w425 {
              tunnel: w424 -> [_ w477]
              tunnel: w423 -> [_ w473]
              tunnel: w422 -> [w470 w476]
              tunnel: w421 -> [w471 w474]
              tunnel: [w470 w475] -> w420
              tunnel: [w471 w472] -> w419
              frame False {
              }
              frame True {
                n176 = Build Array (concatenate)(w476, w477) -> (w475:dbl[][])
                n177 = Build Array (concatenate)(w474, w473) -> (w472:dbl[][])
              }
            }
            n178 = Greater?(x=w434, y=0.1) -> (0:w436:bool)
            n179 = Less?(x=w434, y=-0.1) -> (x < y?=w435:bool)
            n180 = Or(x=w436, y=w435) -> (x .or. y?=w432:bool)
            n181 = local write "Force/Time"(w423) -> ()
            n182 = Reciprocal(x=w464) -> (1/x=w463:dbl)
            n183 = case shown="True" w432 {
              tunnel: w433 -> [_ w480]
              tunnel: w431 -> [_ w478]
              frame False {
              }
              frame True {
                n184 = invoke class="MG17Motor" method="StopImmediate"(reference=w480, error in=w478, "lChanID"=0) -> ()  [unwired: 1 in, 4 out]
              }
            }
            n185 = Multiply(x=w463, y=1000.0) -> (x*y=w462:dbl)
            n186 = Wait (ms)(milliseconds to wait=w462) -> ()  [unwired: 1 out]
          }
          n187 = Build Array (concatenate)(w371, w373) -> (w369:dbl[][])
          n188 = Build Array (concatenate)(w370, w372) -> (w368:dbl[][])
        }
        n189 = Transpose 2D Array(2D array=w313) -> (transposed array=w327:dbl[][])
        n190 = Transpose 2D Array(2D array=w312) -> (transposed array=w328:dbl[][])
        n191 = Transpose 2D Array(2D array=w310) -> (transposed array=w331:dbl[][])
        n192 = Transpose 2D Array(2D array=w311) -> (transposed array=w330:dbl[][])
        n193 = Build Array (concatenate)(w327, w328) -> (w329:dbl[][])
        n194 = Transpose 2D Array(2D array=w329) -> (transposed array=w333:dbl[][])
        n195 = Build Array (concatenate)(w330, w331) -> (w332:dbl[][])
        n196 = local write "Record Data"(w325) -> ()
        n197 = Build Array("Time (s)", "Displacement (mm)", "Force (lbs)") -> (w337:string[])
        n198 = Transpose 2D Array(2D array=w332) -> (transposed array=w334:dbl[][])
        n199 = local write "On/Off"(w319) -> ()
        n200 = Build Array (concatenate)(w333, w334) -> (w335:dbl[][])
        n201 = local write "Record Data"(w319) -> ()
        n202 = local read "Sample Name"() -> (w308:string)
        n203 = call "Sort 2D Array.vim"("index"=0, "2D array"=w335) -> ("sorted 2D array"=w336:dbl[][])  [unwired: 8 in, 1 out]
        n204 = local read "Save Folder Path"() -> (w309:path)
        n205 = Concatenate Strings(w308, ".csv" ("string")) -> (w326:string)
        n206 = Build Path(base path=w309, name or relative path=w326) -> (appended path=w338:path)
        n207 = call-poly <vilib>:"Write Delimited Spreadsheet.vi"("file path (dialog if empty)"=w338, "format (%s)"="%s", "1D data"=w337, "append to file? (new file:F)"=w325, "transpose? (no:F)"=FALSE, "delimiter (\\t)"=",") -> ()  [unwired: 8 in, 2 out]
        n208 = call-poly <vilib>:"Write Delimited Spreadsheet.vi"("file path (dialog if empty)"=w338, "format (%.3f)"="%12.6f", "2D data"=w336, "append to file? (new file:F)"=w319, "transpose? (no:F)"=FALSE ("append to file? (new file:F)"), "delimiter (\\t)"=",") -> ()  [unwired: 8 in, 2 out]
      }
      event "Uniaxial Compression Test": Value Change {
        w616 = FALSE
        w610 = TRUE ("append to file? (new file:F)")
        n209 = event-data() -> ()  [unwired: 1 in, 6 out]
        n210 = call <vilib>:"High Resolution Relative Seconds.vi"() -> ("relative seconds"=w634:dbl)
        n211 = for {
          N: w596 -> [_]
          tunnel: w639 -> [w644]
          tunnel: w637 -> [w686]
          tunnel: w636 -> [w681]
          tunnel: w640 -> [w657]
          tunnel: [w680] -> w638
          tunnel: w635 -> [w670]
          tunnel: w634 -> [w679]
          shift-right: [w672] -> w604
          shift-left: w633 -> [w674]
          shift-right: [w671] -> w603
          shift-left: w632 -> [w673]
          shift-right: [w663] -> w602
          shift-left: w631 -> [w665]
          shift-right: [w662] -> w601
          shift-left: w630 -> [w664]
          shift-right: [w647] -> w597
          shift-left: w641 -> [w658]
          i -> [w697]
          # "Initial Displacement for Down Portion"
          # "Initial Load for Down Portion"
          # "Initial Displacement for Up Portion"
          # "Initial Load for Up Portion"
          n212 = Increment(x=w697) -> (x+1=w643:i32)
          n213 = Negate(x=w644) -> (-x=w645:dbl)
          n214 = local write "Uniaxial Cycles"(w643) -> ()
          n215 = local read "Motor Speed (mm/s)"() -> (w648:dbl)
          n216 = invoke class="MG17Motor" method="SetVelParams"(reference=w658, error in=w657, "lChanID"=0, "fMinVel"=w648, "fAccn"=sgl 1.0, "fMaxVel"=w648) -> (reference out=w656:refnum<k7>, error out=w655:errorcluster)  [unwired: 1 in, 5 out]
          n217 = invoke class="MG17Motor" method="GetPosition"(reference=w656, error in=w655, "lChanID"=0, "pfPosition"=sgl 0.0) -> (reference out=w701:refnum<k7>, error out=w700:errorcluster, "pfPosition"=w696:sgl)  [unwired: 1 in, 2 out]
          n218 = invoke class="MG17Motor" method="SetRelMoveDist"(reference=w701, error in=w700, "lChanID"=0, "fRelDist"=w645) -> (reference out=w705:refnum<k7>, error out=w704:errorcluster)  [unwired: 1 in, 3 out]
          n219 = local read "Exit Loop"() -> (w642:bool)
          n220 = invoke class="MG17Motor" method="MoveRelative"(reference=w705, error in=w704, "lChanID"=0, "bWait"=FALSE) -> (reference out=w646:refnum<k7>, error out=w698:errorcluster)  [unwired: 1 in, 3 out]
          n221 = while {
            tunnel: w698 -> [w850]
            shift-right: [w840] -> _
            shift-left: _ -> [w839]
            tunnel: [w815] -> w654
            tunnel: [w813] -> w653
            tunnel: w686 -> [w838]
            tunnel: w681 -> [w829]
            tunnel: w645 -> [w827]
            tunnel: w696 -> [w826]
            tunnel: w679 -> [w811]
            tunnel: w670 -> [w810]
            shift-right: [w804] -> w675
            shift-left: dbl[][] [] ("Array") -> [w809]
            shift-right: [w803] -> w676
            shift-left: dbl[][] [] ("Array") -> [w808]
            tunnel: w642 -> [w800]
            tunnel: w646 -> [w799]
            stop <- w801 stop-if-true
            # "Safety Factor (80%)"
            # "Lbs"
            n222 = Add(x=w827, y=w826) -> (x+y=w824:dbl)
            n223 = call <vilib>:"High Resolution Relative Seconds.vi"() -> ("relative seconds"=w812:dbl)
            n224 = Tick Count (ms)() -> (millisecond timer value=w840:u32)
            n225 = Subtract(x=w812, y=w811) -> (x-y=w807:dbl)
            n226 = Subtract(x=w840, y=w839) -> (x-y=w843:u32)
            n227 = Unbundle(w838) -> (w837:i32, w836:i32, w835:i32, w834:i32, "new reference"=w832:refnum<k24>, "DeviceHandle"=w831:string, w833:dbl)
            n228 = Divide(x=w843, y=1000) -> (x/y=w841:dbl)
            n229 = invoke class="MG17Motor" method="GetPosition"(reference=w799, error in=w850, "lChanID"=0, "pfPosition"=sgl 0.0) -> (reference out=w815:refnum<k7>, error out=w813:errorcluster, "pfPosition"=w825:sgl)  [unwired: 1 in, 2 out]
            n230 = Subtract(x=w825, y=w824) -> (x-y=w822:dbl)
            n231 = Absolute Value(x=w822) -> (abs(x)=w821:dbl)
            n232 = Less Or Equal?(x=w821, y=0.04) -> (x <= y?=w802:bool)
            n233 = Or(x=w802, y=w800) -> (x .or. y?=w801:bool)
            n234 = Build Array(w825) -> (w797:sgl[])
            n235 = Reciprocal(x=w841) -> (1/x=w798:dbl)
            n236 = while {
              tunnel: [w885] -> _
              tunnel: [w884] -> _
              tunnel: [w883] -> w830
              tunnel: w831 -> [w882]
              tunnel: w832 -> [w881]
              stop <- w880 continue-if-true
              n237 = invoke class="USB_DLL" method="Normal_Data_Request"(reference=w881, "DeviceHandle"=w882) -> (reference out=w885:refnum<k24>, "Normal_Data_Request"=w884:string)  [unwired: 3 in, 3 out]
              n238 = Equal?(x=w884, y="Error") -> (x = y?=w880:bool)
              n239 = Decimal String To Number(string=w884) -> (number=w883:i32)  [unwired: 2 in, 1 out]
            }
            n240 = Build Array (concatenate)(w807, w797) -> (w806:dbl[])
            n241 = local write "Displacement/Time"(w797) -> ()
            n242 = local write "1/x 3"(w798) -> ()
            n243 = xnode "Formula"("Get_Offset_Value"=w837, "Get_Offset_Load"=w836, "Get_Fullscale_Value"=w835, "Get_Fullscale_Load"=w834, "Get_Decimal_Point"=w833, "Normal_Data_Request"=w830) -> ("Result"=w816:dbl)  [unwired: 1 in, 1 out]
            n244 = Subtract(x=w816, y=w829) -> (x-y=w828:dbl)
            n245 = local read "Sampling Rate (Hz)"() -> (w846:dbl)
            n246 = Build Array(w828) -> (w805:dbl[])
            n247 = case shown="True" w810 {
              tunnel: w809 -> [w852 w857]
              tunnel: w808 -> [w851 w856]
              tunnel: w806 -> [_ w858]
              tunnel: w805 -> [_ w855]
              tunnel: [w851 w854] -> w803
              tunnel: [w852 w853] -> w804
              frame False {
              }
              frame True {
                n248 = Build Array (concatenate)(w857, w858) -> (w853:dbl[][])
                n249 = Build Array (concatenate)(w856, w855) -> (w854:dbl[][])
              }
            }
            n250 = Greater?(x=w816, y=0.1) -> (0:w818:bool)
            n251 = Less?(x=w816, y=-0.1) -> (x < y?=w817:bool)
            n252 = Or(x=w818, y=w817) -> (x .or. y?=w814:bool)
            n253 = local write "Force/Time"(w805) -> ()
            n254 = Reciprocal(x=w846) -> (1/x=w845:dbl)
            n255 = case shown="True" w814 {
              tunnel: w815 -> [_ w861]
              tunnel: w813 -> [_ w859]
              frame False {
              }
              frame True {
                n256 = invoke class="MG17Motor" method="StopImmediate"(reference=w861, error in=w859, "lChanID"=0) -> ()  [unwired: 1 in, 4 out]
              }
            }
            n257 = Multiply(x=w845, y=1000.0) -> (x*y=w844:dbl)
            n258 = Wait (ms)(milliseconds to wait=w844) -> ()  [unwired: 1 out]
          }
          n259 = invoke class="MG17Motor" method="SetVelParams"(reference=w654, error in=w653, "lChanID"=0, "fMinVel"=w648, "fAccn"=sgl 1.0, "fMaxVel"=w648) -> (reference out=w652:refnum<k7>, error out=w651:errorcluster)  [unwired: 1 in, 5 out]
          n260 = invoke class="MG17Motor" method="GetPosition"(reference=w652, error in=w651, "lChanID"=0, "pfPosition"=sgl 0.0) -> (reference out=w690:refnum<k7>, error out=w689:errorcluster, "pfPosition"=w683:sgl)  [unwired: 1 in, 2 out]
          n261 = Build Array (concatenate)(w674, w675) -> (w672:dbl[][])
          n262 = Build Array (concatenate)(w673, w676) -> (w671:dbl[][])
          n263 = invoke class="MG17Motor" method="SetRelMoveDist"(reference=w690, error in=w689, "lChanID"=0, "fRelDist"=w644) -> (reference out=w694:refnum<k7>, error out=w693:errorcluster, "fRelDist"=w682:sgl)  [unwired: 1 in, 2 out]
          n264 = invoke class="MG17Motor" method="MoveRelative"(reference=w694, error in=w693, "lChanID"=0, "bWait"=FALSE) -> (reference out=w685:refnum<k7>, error out=w684:errorcluster)  [unwired: 1 in, 3 out]
          n265 = while {
            tunnel: w685 -> [w760]
            tunnel: w684 -> [w759]
            shift-right: [w749] -> _
            shift-left: _ -> [w748]
            tunnel: [w724] -> w647
            tunnel: [w722] -> w680
            tunnel: w686 -> [w747]
            tunnel: w681 -> [w738]
            tunnel: w682 -> [w736]
            tunnel: w683 -> [w735]
            tunnel: w679 -> [w719]
            tunnel: w670 -> [w716]
            shift-right: [w711] -> w667
            shift-left: dbl[][] [] ("Array") -> [w713]
            shift-right: [w710] -> w666
            shift-left: dbl[][] [] ("Array") -> [w712]
            tunnel: w642 -> [w708]
            stop <- w707 stop-if-true
            # "Safety Factor (80%)"
            # "Grams"
            n266 = Add(x=w736, y=w735) -> (x+y=w733:sgl)
            n267 = call <vilib>:"High Resolution Relative Seconds.vi"() -> ("relative seconds"=w720:dbl)
            n268 = Tick Count (ms)() -> (millisecond timer value=w749:u32)
            n269 = Subtract(x=w720, y=w719) -> (x-y=w718:dbl)
            n270 = Subtract(x=w749, y=w748) -> (x-y=w752:u32)
            n271 = Unbundle(w747) -> (w746:i32, w745:i32, w744:i32, w743:i32, "new reference"=w741:refnum<k24>, "DeviceHandle"=w740:string, w742:dbl)
            n272 = Divide(x=w752, y=1000) -> (x/y=w750:dbl)
            n273 = invoke class="MG17Motor" method="GetPosition"(reference=w760, error in=w759, "lChanID"=0, "pfPosition"=sgl 0.0) -> (reference out=w724:refnum<k7>, error out=w722:errorcluster, "pfPosition"=w734:sgl)  [unwired: 1 in, 2 out]
            n274 = Subtract(x=w734, y=w733) -> (x-y=w731:sgl)
            n275 = Absolute Value(x=w731) -> (abs(x)=w730:sgl)
            n276 = Less Or Equal?(x=w730, y=0.04) -> (x <= y?=w709:bool)
            n277 = Or(x=w709, y=w708) -> (x .or. y?=w707:bool)
            n278 = Build Array(w734) -> (w717:sgl[])
            n279 = Build Array (concatenate)(w718, w717) -> (w715:dbl[])
            n280 = Reciprocal(x=w750) -> (1/x=w721:dbl)
            n281 = while {
              tunnel: [w795] -> _
              tunnel: [w794] -> _
              tunnel: [w793] -> w739
              tunnel: w740 -> [w792]
              tunnel: w741 -> [w791]
              stop <- w790 continue-if-true
              n282 = invoke class="USB_DLL" method="Normal_Data_Request"(reference=w791, "DeviceHandle"=w792) -> (reference out=w795:refnum<k24>, "Normal_Data_Request"=w794:string)  [unwired: 3 in, 3 out]
              n283 = Equal?(x=w794, y="Error") -> (x = y?=w790:bool)
              n284 = Decimal String To Number(string=w794) -> (number=w793:i32)  [unwired: 2 in, 1 out]
            }
            n285 = local write "1/x 3"(w721) -> ()
            n286 = xnode "Formula"("Get_Offset_Value"=w746, "Get_Offset_Load"=w745, "Get_Fullscale_Value"=w744, "Get_Fullscale_Load"=w743, "Get_Decimal_Point"=w742, "Normal_Data_Request"=w739) -> ("Result"=w725:dbl)  [unwired: 1 in, 1 out]
            n287 = local write "Displacement/Time"(w717) -> ()
            n288 = Subtract(x=w725, y=w738) -> (x-y=w737:dbl)
            n289 = local read "Sampling Rate (Hz)"() -> (w755:dbl)
            n290 = Build Array(w737) -> (w714:dbl[])
            n291 = case shown="True" w716 {
              tunnel: w715 -> [_ w768]
              tunnel: w714 -> [_ w764]
              tunnel: w713 -> [w761 w767]
              tunnel: w712 -> [w762 w765]
              tunnel: [w761 w766] -> w711
              tunnel: [w762 w763] -> w710
              frame False {
              }
              frame True {
                n292 = Build Array (concatenate)(w767, w768) -> (w766:dbl[][])
                n293 = Build Array (concatenate)(w765, w764) -> (w763:dbl[][])
              }
            }
            n294 = Greater?(x=w725, y=0.1) -> (0:w727:bool)
            n295 = Less?(x=w725, y=-0.1) -> (x < y?=w726:bool)
            n296 = Or(x=w727, y=w726) -> (x .or. y?=w723:bool)
            n297 = local write "Force/Time"(w714) -> ()
            n298 = Reciprocal(x=w755) -> (1/x=w754:dbl)
            n299 = case shown="True" w723 {
              tunnel: w724 -> [_ w771]
              tunnel: w722 -> [_ w769]
              frame False {
              }
              frame True {
                n300 = invoke class="MG17Motor" method="StopImmediate"(reference=w771, error in=w769, "lChanID"=0) -> ()  [unwired: 1 in, 4 out]
              }
            }
            n301 = Multiply(x=w754, y=1000.0) -> (x*y=w753:dbl)
            n302 = Wait (ms)(milliseconds to wait=w753) -> ()  [unwired: 1 out]
          }
          n303 = Build Array (concatenate)(w665, w667) -> (w663:dbl[][])
          n304 = Build Array (concatenate)(w664, w666) -> (w662:dbl[][])
        }
        n305 = Transpose 2D Array(2D array=w604) -> (transposed array=w618:dbl[][])
        n306 = Transpose 2D Array(2D array=w603) -> (transposed array=w619:dbl[][])
        n307 = Transpose 2D Array(2D array=w601) -> (transposed array=w622:dbl[][])
        n308 = Transpose 2D Array(2D array=w602) -> (transposed array=w621:dbl[][])
        n309 = Build Array (concatenate)(w618, w619) -> (w620:dbl[][])
        n310 = Transpose 2D Array(2D array=w620) -> (transposed array=w624:dbl[][])
        n311 = Build Array (concatenate)(w621, w622) -> (w623:dbl[][])
        n312 = local write "Record Data"(w616) -> ()
        n313 = Build Array("Time (s)", "Displacement (mm)", "Force (lbs)") -> (w628:string[])
        n314 = Transpose 2D Array(2D array=w623) -> (transposed array=w625:dbl[][])
        n315 = local write "On/Off"(w610) -> ()
        n316 = Build Array (concatenate)(w624, w625) -> (w626:dbl[][])
        n317 = local write "Record Data"(w610) -> ()
        n318 = local read "Sample Name"() -> (w599:string)
        n319 = call "Sort 2D Array.vim"("index"=0, "2D array"=w626) -> ("sorted 2D array"=w627:dbl[][])  [unwired: 8 in, 1 out]
        n320 = local read "Save Folder Path"() -> (w600:path)
        n321 = Concatenate Strings(w599, ".csv" ("string")) -> (w617:string)
        n322 = Build Path(base path=w600, name or relative path=w617) -> (appended path=w629:path)
        n323 = call-poly <vilib>:"Write Delimited Spreadsheet.vi"("file path (dialog if empty)"=w629, "format (%s)"="%s", "1D data"=w628, "append to file? (new file:F)"=w616, "transpose? (no:F)"=FALSE, "delimiter (\\t)"=",") -> ()  [unwired: 8 in, 2 out]
        n324 = call-poly <vilib>:"Write Delimited Spreadsheet.vi"("file path (dialog if empty)"=w629, "format (%.3f)"="%12.6f", "2D data"=w627, "append to file? (new file:F)"=w610, "transpose? (no:F)"=FALSE ("append to file? (new file:F)"), "delimiter (\\t)"=",") -> ()  [unwired: 8 in, 2 out]
      }
      event "Home Z Motor": Value Change {
        n325 = event-data() -> ()  [unwired: 1 in, 6 out]
        n326 = call "Prompt User for Input2"() -> ("OK"=w889:bool)  [unwired: 18 in, 1 out]
        n327 = case shown="True" w889 {
          tunnel: w891 -> [w893 w897]
          tunnel: w890 -> [w892 w896]
          tunnel: [w893 w895] -> w888
          tunnel: [w892 w894] -> w887
          frame False {
          }
          frame True {
            n328 = invoke class="MG17Motor" method="MoveHome"(reference=w897, error in=w896, "lChanID"=0, "bWait"=FALSE) -> (reference out=w895:refnum<k7>, error out=w894:errorcluster)  [unwired: 1 in, 3 out]
          }
        }
      }
      event "Up": Value Change {
        n329 = event-data() -> ()  [unwired: 1 in, 6 out]
        n330 = invoke class="MG17Motor" method="SetJogVelParams"(reference=w914, error in=w913, "lChanID"=0, "fMinVel"=w910, "fAccn"=sgl 0.0, "fMaxVel"=w910) -> (reference out=w909:refnum<k7>, error out=w908:errorcluster)  [unwired: 1 in, 5 out]
        n331 = invoke class="MG17Motor" method="SetJogStepSize"(reference=w909, error in=w908, "lChanID"=0, "fStepSize"=w906) -> (reference out=w905:refnum<k7>, error out=w904:errorcluster)  [unwired: 1 in, 3 out]
        n332 = invoke class="MG17Motor" method="MoveJog"(reference=w905, error in=w904, "lChanID"=0, "lJogDir"=1) -> (reference out=w901:refnum<k7>, error out=w900:errorcluster)  [unwired: 1 in, 3 out]
      }
      event "Down": Value Change {
        n333 = event-data() -> ()  [unwired: 1 in, 6 out]
        n334 = invoke class="MG17Motor" method="SetJogVelParams"(reference=w929, error in=w928, "lChanID"=0, "fMinVel"=w925, "fAccn"=sgl 1.0, "fMaxVel"=w925) -> (reference out=w924:refnum<k7>, error out=w923:errorcluster)  [unwired: 1 in, 5 out]
        n335 = invoke class="MG17Motor" method="SetJogStepSize"(reference=w924, error in=w923, "lChanID"=0, "fStepSize"=w921) -> (reference out=w920:refnum<k7>, error out=w919:errorcluster)  [unwired: 1 in, 3 out]
        n336 = invoke class="MG17Motor" method="MoveJog"(reference=w920, error in=w919, "lChanID"=0, "lJogDir"=2) -> (reference out=w916:refnum<k7>, error out=w915:errorcluster)  [unwired: 1 in, 3 out]
      }
      event "1 Step Test Button": Value Change {
        # "Initial Angle"
        # "Initial Loads"
        n337 = event-data() -> ()  [unwired: 1 in, 6 out]
        n338 = flat-sequence {
          tunnel: w962 -> [w1044]
          tunnel: w972 -> [w1045]
          tunnel: w973 -> [w1046]
          tunnel: w974 -> [w1047]
          tunnel: w982 -> [w1048]
          tunnel: [w1048] -> w943
          tunnel: [w1047] -> w941
          tunnel: [w1046] -> w939
          tunnel: [w1045] -> w937
          tunnel: [w1044] -> w935
          tunnel: w955 -> [w1028]
          tunnel: w954 -> [w1036]
          tunnel: w953 -> [w1035]
          tunnel: [w1038] -> w933
          tunnel: [w1037] -> w931
          tunnel: w952 -> [w1030]
          tunnel: w943 -> [w1055]
          tunnel: [w1055] -> w942
          tunnel: w941 -> [w1054]
          tunnel: [w1054] -> w940
          tunnel: w939 -> [w1053]
          tunnel: [w1053] -> w938
          tunnel: w937 -> [w1052]
          tunnel: [w1052] -> w936
          tunnel: w935 -> [w1051]
          tunnel: [w1051] -> w934
          tunnel: w933 -> [w1050]
          tunnel: [w1050] -> w932
          tunnel: w931 -> [w1049]
          tunnel: [w1049] -> w930
          tunnel: [w1069] -> w981
          tunnel: [w1068] -> w980
          tunnel: w942 -> [w1072]
          tunnel: w940 -> [w1066]
          tunnel: w938 -> [w1065]
          tunnel: w936 -> [w1063]
          tunnel: w934 -> [w1059]
          tunnel: w932 -> [w1057]
          tunnel: w930 -> [w1056]
          tunnel: [w1057] -> w949
          tunnel: [w1056] -> w948
          frame #0 {
            n339 = invoke class="MG17Motor" method="SetVelParams"(reference=w1036, error in=w1035, "lChanID"=0, "fMinVel"=sgl 0.0, "fAccn"=sgl 1.0, "fMaxVel"=w1030) -> (reference out=w1034:refnum<k7>, error out=w1033:errorcluster)  [unwired: 1 in, 5 out]
            n340 = Negate(x=w1028) -> (-x=w1027:dbl)
            n341 = invoke class="MG17Motor" method="SetRelMoveDist"(reference=w1034, error in=w1033, "lChanID"=0, "fRelDist"=w1027) -> (reference out=w1042:refnum<k7>, error out=w1041:errorcluster)  [unwired: 1 in, 3 out]
            n342 = invoke class="MG17Motor" method="MoveRelative"(reference=w1042, error in=w1041, "lChanID"=0, "bWait"=FALSE) -> (reference out=w1038:refnum<k7>, error out=w1037:errorcluster)  [unwired: 1 in, 3 out]
          }
          frame #1 {
          }
          frame #2 {
            w1060 = u16 4 items=["device units", "microns/s, microns/s^2", "mm/s, mm/s^2", "inches/s, inches/s^2", "degrees/s, degrees/s^2"] ("Units (0: data)")
            w1071 = u16 0 items=["relative", "absolute"] ("Movement Type (0: relative)")
            n343 = local read "Speed (Deg/s)"() -> (w1067:dbl)
            n344 = call "Set Speed and Acceleration.vi"("Units (0: data)"=w1060, "New Speed (0)"=w1067, "error in (no error)"=w1065, "Device and Axis"="01", "Microstep Size (0)"=w1063, "VISA resource name"=w1066) -> ("error out"=w1062:errorcluster, "VISA resource name out"=w1061:refnum<visa-resource-name>)  [unwired: 4 in]
            n345 = Negate(x=w1059) -> (-x=w1058:dbl)
            n346 = call "Move.vi"("Units (0: microsteps)"=w1072, "Movement Type (0: relative)"=w1071, "Move Distance (0)"=w1058, "error in (no error)"=w1062, "Device and Axis"="01", "Microstep Size (0)"=w1063, "VISA resource name"=w1061) -> ("error out"=w1068:errorcluster, "VISA resource name out"=w1069:refnum<visa-resource-name>)  [unwired: 3 in]
          }
        }
        n347 = call <vilib>:"High Resolution Relative Seconds.vi"() -> ("relative seconds"=w961:dbl)
        n348 = while {
          tunnel: w981 -> [w1137]
          tunnel: w980 -> [w1136]
          tunnel: [w1113] -> w978
          tunnel: [w1112] -> w979
          tunnel: w977 -> [w1075]
          tunnel: w976 -> [w1111]
          shift-right: [w1101] -> _
          shift-left: _ -> [w1128]
          tunnel: w975 -> [w1123]
          tunnel: w971 -> [w1105]
          shift-right: [w1108] -> w967
          shift-left: dbl[][] [] ("Array") -> [w1106]
          shift-right: [w1102] -> w966
          shift-left: dbl[][] [] ("Array") -> [w1103]
          tunnel: w961 -> [w1099]
          shift-right: [w1094] -> w959
          shift-left: w960 -> [w1094]
          tunnel: w956 -> [w1085]
          stop <- w1124 stop-if-true
          w1135 = u16 4 items=["microsteps", "microns", "millimeters", "inches", "degrees"] ("Units (0: microsteps)")
          n349 = call <vilib>:"High Resolution Relative Seconds.vi"() -> ("relative seconds"=w1096:dbl)
          n350 = Tick Count (ms)() -> (millisecond timer value=w1101:u32)
          n351 = Subtract(x=w1096, y=w1099) -> (x-y=w1098:dbl)
          n352 = Subtract(x=w1101, y=w1128) -> (x-y=w1127:u32)
          n353 = Divide(x=w1127, y=u32 1000 ("millisecond timer value")) -> (x/y=w1125:dbl)
          n354 = Unbundle(w1085) -> (w1084:i32, w1083:i32, w1082:i32, w1081:i32, "new reference"=w1079:refnum<k24>, "DeviceHandle"=w1078:string, w1080:dbl)
          n355 = Unbundle(w1123) -> (w1122:i32, w1121:i32, w1120:i32, w1119:i32, "new reference"=w1092:refnum<k24>, "DeviceHandle"=w1093:string, w1118:dbl)
          n356 = call "Read Current Position.vi"("Units (0: microsteps)"=w1135, "error in (no error)"=w1136, "Device and Axis"="01", "Microstep Size (0)"=0.000234375, "VISA resource name"=w1137) -> ("error out"=w1132:errorcluster, "Position"=w1129:dbl, "VISA resource name out"=w1131:refnum<visa-resource-name>)  [unwired: 4 in]
          n357 = Build Array(w1129) -> (w1095:dbl[])
          n358 = call "Check for Idle.vi"("error in (no error)"=w1132, "Device and Axis"="01", "VISA resource name"=w1131) -> ("error out"=w1113:errorcluster, "Idle"=w1124:bool, "VISA resource name out"=w1112:refnum<visa-resource-name>)  [unwired: 6 in]
          n359 = Negate(x=w1095) -> (-x=w1090:dbl[])
          n360 = Build Array (concatenate)(w1098, w1090) -> (w1107:dbl[])
          n361 = while {
            tunnel: [w1169] -> _
            tunnel: [w1168] -> _
            tunnel: [w1167] -> w1091
            tunnel: w1093 -> [w1166]
            tunnel: w1092 -> [w1165]
            tunnel: [w1163] -> _
            tunnel: [w1162] -> w1077
            tunnel: [w1161] -> _
            tunnel: w1079 -> [w1160]
            tunnel: w1078 -> [w1159]
            stop <- w1156 continue-if-true
            n362 = invoke class="USB_DLL" method="Normal_Data_Request"(reference=w1165, "DeviceHandle"=w1166) -> (reference out=w1169:refnum<k24>, "Normal_Data_Request"=w1168:string)  [unwired: 3 in, 3 out]
            n363 = invoke class="USB_DLL" method="Normal_Data_Request"(reference=w1160, "DeviceHandle"=w1159) -> (reference out=w1161:refnum<k24>, "Normal_Data_Request"=w1163:string)  [unwired: 3 in, 3 out]
            n364 = Equal?(x=w1168, y="Error") -> (x = y?=w1158:bool)
            n365 = Equal?(x=w1163, y="Error") -> (x = y?=w1157:bool)
            n366 = Or(x=w1158, y=w1157) -> (x .or. y?=w1156:bool)
            n367 = Decimal String To Number(string=w1168) -> (number=w1167:i32)  [unwired: 2 in, 1 out]
            n368 = Decimal String To Number(string=w1163) -> (number=w1162:i32)  [unwired: 2 in, 1 out]
          }
          n369 = Reciprocal(x=w1125) -> (1/x=w1097:dbl)
          n370 = local write "Angle/Time"(w1090) -> ()
          n371 = local write "1/x 2"(w1097) -> ()
          n372 = xnode "Formula"("Get_Offset_Value"=w1084, "Get_Offset_Load"=w1083, "Get_Fullscale_Value"=w1082, "Get_Fullscale_Load"=w1081, "Get_Decimal_Point"=w1080, "Normal_Data_Request"=w1077) -> ("Result"=w1076:dbl)  [unwired: 1 in, 1 out]
          n373 = xnode "Formula"("Get_Offset_Value"=w1122, "Get_Offset_Load"=w1121, "Get_Fullscale_Value"=w1120, "Get_Fullscale_Load"=w1119, "Get_Decimal_Point"=w1118, "Normal_Data_Request"=w1091) -> ("Result"=w1109:dbl)  [unwired: 1 in, 1 out]
          n374 = Subtract(x=w1109, y=w1111) -> (x-y=w1110:dbl)
          n375 = Subtract(x=w1076, y=w1075) -> (x-y=w1074:dbl)
          n376 = Greater?(x=w1109, y=11.2) -> (0:w1115:bool)
          n377 = Less?(x=w1109, y=-11.2) -> (x < y?=w1114:bool)
          n378 = Build Array(w1110) -> (w1100:dbl[])
          n379 = Build Array(w1074) -> (w1073:dbl[])
          n380 = Or(x=w1115, y=w1114) -> ()  [unwired: 1 out]
          n381 = local write "Torque/Time"(w1100) -> ()
          n382 = local read "Sampling Rate (Hz)"() -> (w1088:dbl)
          n383 = local write "Force/Time"(w1073) -> ()
          n384 = Build Array (concatenate)(w1100, w1073) -> (w1104:dbl[])
          n385 = case shown="True" w1105 {
            tunnel: [w1172 w1178] -> w1108
            tunnel: w1107 -> [_ w1177]
            tunnel: w1106 -> [w1172 w1176]
            tunnel: w1104 -> [_ w1175]
            tunnel: w1103 -> [w1171 w1174]
            tunnel: [w1171 w1173] -> w1102
            frame False {
            }
            frame True {
              n386 = Build Array (concatenate)(w1176, w1177) -> (w1178:dbl[][])
              n387 = Build Array (concatenate)(w1174, w1175) -> (w1173:dbl[][])
            }
          }
          n388 = Reciprocal(x=w1088) -> (1/x=w1087:dbl)
          n389 = Multiply(x=w1087, y=1000.0) -> (x*y=w1086:dbl)
          n390 = Wait (ms)(milliseconds to wait=w1086) -> ()  [unwired: 1 out]
        }
        n391 = Build Array (concatenate)(w968, w967) -> (w958:dbl[][])
        n392 = Build Array (concatenate)(w965, w966) -> (w957:dbl[][])
        n393 = flat-sequence {
          tunnel: w957 -> [w999]
          tunnel: w958 -> [w1000]
          tunnel: [w1000] -> w951
          tunnel: [w999] -> w950
          tunnel: w949 -> [w988]
          tunnel: w948 -> [w987]
          tunnel: [w984] -> w947
          tunnel: [w983] -> w946
          tunnel: w951 -> [w1010]
          tunnel: w950 -> [w1009]
          tunnel: w947 -> [w1002]
          tunnel: w946 -> [w1001]
          tunnel: [w1002] -> w945
          tunnel: [w1001] -> w944
          frame #0 {
            n394 = local read "Motor Speed (mm/s)"() -> (w986:dbl)
            n395 = invoke class="MG17Motor" method="SetVelParams"(reference=w988, error in=w987, "lChanID"=0, "fMinVel"=sgl 0.0, "fAccn"=sgl 1.0, "fMaxVel"=w986) -> (reference out=w993:refnum<k7>, error out=w992:errorcluster)  [unwired: 1 in, 5 out]
            n396 = local read "Compression (mm)"() -> (w985:dbl)
            n397 = invoke class="MG17Motor" method="SetRelMoveDist"(reference=w993, error in=w992, "lChanID"=0, "fRelDist"=w985) -> (reference out=w997:refnum<k7>, error out=w996:errorcluster)  [unwired: 1 in, 3 out]
            n398 = invoke class="MG17Motor" method="MoveRelative"(reference=w997, error in=w996, "lChanID"=0, "bWait"=FALSE) -> (reference out=w984:refnum<k7>, error out=w983:errorcluster)  [unwired: 1 in, 3 out]
          }
          frame #1 {
            w1021 = FALSE
            w1015 = TRUE ("append to file? (new file:F)")
            n399 = Transpose 2D Array(2D array=w1010) -> (transposed array=w1023:dbl[][])
            n400 = Transpose 2D Array(2D array=w1009) -> (transposed array=w1024:dbl[][])
            n401 = Build Array (concatenate)(w1023, w1024) -> (w1005:dbl[][])
            n402 = local write "Record Data"(w1021) -> ()
            n403 = Transpose 2D Array(2D array=w1005) -> (transposed array=w1004:dbl[][])
            n404 = Build Array("Time (s)", "Angle (Degrees)", "Torque (in-oz)", "Force (lbs)") -> (w1025:string[])
            n405 = local write "On/Off"(w1015) -> ()
            n406 = local write "Record Data"(w1015) -> ()
            n407 = local read "Sample Name"() -> (w1006:string)
            n408 = local read "Save Folder Path"() -> (w1007:path)
            n409 = Concatenate Strings(w1006, ".csv" ("string")) -> (w1022:string)
            n410 = Build Path(base path=w1007, name or relative path=w1022) -> (appended path=w1026:path)
            n411 = call-poly <vilib>:"Write Delimited Spreadsheet.vi"("file path (dialog if empty)"=w1026, "format (%s)"="%s", "1D data"=w1025, "append to file? (new file:F)"=w1021, "transpose? (no:F)"=FALSE, "delimiter (\\t)"=",") -> ()  [unwired: 8 in, 2 out]
            n412 = call-poly <vilib>:"Write Delimited Spreadsheet.vi"("file path (dialog if empty)"=w1026, "format (%.3f)"="%12.6f", "2D data"=w1004, "append to file? (new file:F)"=w1015, "transpose? (no:F)"=FALSE ("append to file? (new file:F)"), "delimiter (\\t)"=",") -> ()  [unwired: 8 in, 2 out]
          }
        }
      }
      event "Cyclic Test Button": Value Change {
        w1215 = FALSE
        w1203 = TRUE ("append to file? (new file:F)")
        n413 = event-data() -> ()  [unwired: 1 in, 6 out]
        n414 = call <vilib>:"High Resolution Relative Seconds.vi"() -> ("relative seconds"=w1231:dbl)
        n415 = for {
          N: w1249 -> [_]
          shift-right: [w1299] -> w1244
          shift-left: w1243 -> [w1293]
          tunnel: w1247 -> [w1295]
          tunnel: w1248 -> [w1289]
          tunnel: w1247 -> [w1309]
          tunnel: w1246 -> [w1307]
          shift-right: [w1298] -> w1245
          shift-left: _ -> [_]
          tunnel: w1241 -> [w1272]
          tunnel: w1238 -> [w1281]
          tunnel: w1238 -> [w1280]
          shift-right: [w1277] -> _
          shift-left: 0 -> [w1279]
          tunnel: w1239 -> [w1275]
          tunnel: w1237 -> [w1276]
          tunnel: w1237 -> [w1274]
          tunnel: w1236 -> [w1270]
          shift-right: [w1265] -> w1204
          shift-left: w1235 -> [w1258]
          shift-right: [w1264] -> w1205
          shift-left: w1234 -> [w1257]
          shift-right: [w1254] -> w1206
          shift-left: w1233 -> [w1256]
          shift-right: [w1253] -> w1207
          shift-left: w1232 -> [w1255]
          tunnel: w1231 -> [w1252]
          tunnel: w1198 -> [w1250]
          i -> [w1297]
          w1302 = u16 0 items=["relative", "absolute"] ("Movement Type (0: relative)")
          w1303 = u16 4 items=["microsteps", "microns", "millimeters", "inches", "degrees"] ("Units (0: microsteps)")
          w1283 = "01" ("Device and Axis")
          w1282 = 0.000234375
          w1284 = u16 4 items=["device units", "microns/s, microns/s^2", "mm/s, mm/s^2", "inches/s, inches/s^2", "degrees/s, degrees/s^2"] ("Units (0: data)")
          w1306 = u16 0 items=["relative", "absolute"] ("Movement Type (0: relative)")
          w1292 = u16 4 items=["device units", "microns/s, microns/s^2", "mm/s, mm/s^2", "inches/s, inches/s^2", "degrees/s, degrees/s^2"] ("Units (0: data)")
          # "Initial Angle"
          # "Initial Loads"
          # "Initial Angle for CCW Portion"
          # "Initial Loads for CCW Portion"
          n416 = Increment(x=w1297) -> (x+1=→"Current Cycle":i32)
          n417 = local read "Speed (Deg/s)"() -> (w1273:dbl)
          n418 = call "Set Speed and Acceleration.vi"("Units (0: data)"=w1292, "New Speed (0)"=w1273, "error in (no error)"=w1293, "Device and Axis"="01", "Microstep Size (0)"=w1295, "VISA resource name"=w1289) -> ("error out"=w1291:errorcluster, "VISA resource name out"=w1290:refnum<visa-resource-name>)  [unwired: 4 in]
          n419 = call "Move.vi"("Units (0: microsteps)"=w1307, "Movement Type (0: relative)"=w1306, "Move Distance (0)"=w1272, "error in (no error)"=w1291, "Device and Axis"="01", "Microstep Size (0)"=w1309, "VISA resource name"=w1290) -> ("error out"=w1304:errorcluster, "VISA resource name out"=w1305:refnum<visa-resource-name>)  [unwired: 3 in]
          n420 = while {
            tunnel: w1305 -> [w1510]
            tunnel: w1304 -> [w1468]
            tunnel: [w1486] -> w1288
            tunnel: [w1487] -> w1287
            tunnel: w1281 -> [w1454]
            shift-right: [w1479] -> w1278
            shift-left: w1279 -> [w1504]
            tunnel: w1275 -> [w1500]
            tunnel: w1276 -> [w1485]
            tunnel: w1270 -> [w1469]
            shift-right: [w1473] -> w1267
            shift-left: dbl[][] [] ("Array") -> [w1475]
            shift-right: [w1472] -> w1266
            shift-left: dbl[][] [] ("Array") -> [w1474]
            tunnel: [w1469] -> w1261
            tunnel: w1252 -> [w1465]
            tunnel: [w1465] -> w1251
            tunnel: w1250 -> [w1463]
            stop <- w1505 stop-if-true
            w1513 = u16 4 items=["microsteps", "microns", "millimeters", "inches", "degrees"] ("Units (0: microsteps)")
            # "Grams"
            n421 = call <vilib>:"High Resolution Relative Seconds.vi"() -> ("relative seconds"=w1467:dbl)
            n422 = Tick Count (ms)() -> (millisecond timer value=w1479:u32)
            n423 = Unbundle(w1500) -> (w1499:i32, w1498:i32, w1497:i32, w1496:i32, "new reference"=w1493:refnum<k24>, "DeviceHandle"=w1492:string, w1495:dbl)
            n424 = Unbundle(w1463) -> (w1460:i32, w1459:i32, w1458:i32, w1457:i32, "new reference"=w1461:refnum<k24>, "DeviceHandle"=w1462:string, w1456:dbl)
            n425 = Subtract(x=w1479, y=w1504) -> (x-y=w1503:u32)
            n426 = Subtract(x=w1467, y=w1465) -> (x-y=w1466:dbl)
            n427 = Divide(x=w1503, y=1000) -> (x/y=w1501:dbl)
            n428 = while {
              tunnel: [w1553] -> w1494
              tunnel: w1493 -> [w1552]
              tunnel: [w1551] -> _
              tunnel: w1492 -> [w1550]
              tunnel: [w1549] -> _
              tunnel: [w1547] -> _
              tunnel: [w1546] -> _
              tunnel: w1462 -> [w1542]
              tunnel: w1461 -> [w1541]
              tunnel: [w1540] -> w1455
              stop <- w1543 continue-if-true
              n429 = invoke class="USB_DLL" method="Normal_Data_Request"(reference=w1541, "DeviceHandle"=w1542) -> (reference out=w1546:refnum<k24>, "Normal_Data_Request"=w1547:string)  [unwired: 3 in, 3 out]
              n430 = invoke class="USB_DLL" method="Normal_Data_Request"(reference=w1552, "DeviceHandle"=w1550) -> (reference out=w1551:refnum<k24>, "Normal_Data_Request"=w1549:string)  [unwired: 3 in, 3 out]
              n431 = Equal?(x=w1547, y="Error") -> (x = y?=w1544:bool)
              n432 = Equal?(x=w1549, y="Error") -> (x = y?=w1545:bool)
              n433 = Or(x=w1545, y=w1544) -> (x .or. y?=w1543:bool)
              n434 = Decimal String To Number(string=w1547) -> (number=w1540:i32)  [unwired: 2 in, 1 out]
              n435 = Decimal String To Number(string=w1549) -> (number=w1553:i32)  [unwired: 2 in, 1 out]
            }
            n436 = Reciprocal(x=w1501) -> (1/x=→"1/x":dbl)
            n437 = xnode "Formula"("Get_Offset_Value"=w1460, "Get_Offset_Load"=w1459, "Get_Fullscale_Value"=w1458, "Get_Fullscale_Load"=w1457, "Get_Decimal_Point"=w1456, "Normal_Data_Request"=w1455) -> ("Result"=w1447:dbl)  [unwired: 1 in, 1 out]
            n438 = xnode "Formula"("Get_Offset_Value"=w1499, "Get_Offset_Load"=w1498, "Get_Fullscale_Value"=w1497, "Get_Fullscale_Load"=w1496, "Get_Decimal_Point"=w1495, "Normal_Data_Request"=w1494) -> ("Result"=w1470:dbl)  [unwired: 1 in, 1 out]
            n439 = Greater?(x=w1447, y=800.0) -> (0:w1449:bool)
            n440 = Less?(x=w1447, y=-800.0) -> (x < y?=w1448:bool)
            n441 = Or(x=w1449, y=w1448) -> (x .or. y?=w1446:bool)
            n442 = call "Read Current Position.vi"("Units (0: microsteps)"=w1513, "error in (no error)"=w1468, "Device and Axis"="01", "Microstep Size (0)"=0.000234375, "VISA resource name"=w1510) -> ("error out"=w1487:errorcluster, "Position"=w1508:dbl, "VISA resource name out"=w1486:refnum<visa-resource-name>)  [unwired: 4 in]
            n443 = call "Check for Idle.vi"("error in (no error)"=w1468, "Device and Axis"="01", "VISA resource name"=w1510) -> ("Idle"=w1507:bool)  [unwired: 6 in, 2 out]
            n444 = Build Array(w1507) -> (w1506:bool[])
            n445 = Build Array(w1508) -> (w1464:dbl[])
            "Angle/Time" <- w1464
            n446 = Build Array (concatenate)(w1466, w1464) -> (w1476:dbl[])
            n447 = Subtract(x=w1470, y=w1485) -> (x-y=w1484:dbl)
            n448 = Subtract(x=w1447, y=w1454) -> (x-y=w1453:dbl)
            n449 = Greater?(x=w1470, y=11.2) -> (0:w1489:bool)
            n450 = Less?(x=w1470, y=-11.2) -> (x < y?=w1488:bool)
            n451 = And Array Elements(Boolean array=w1506) -> (logical AND=w1505:bool)
            n452 = Build Array(w1484) -> (w1471:dbl[])
            "Torque/Time" <- w1471
            n453 = Build Array(w1453) -> (w1452:dbl[])
            "Force/Time" <- w1452
            n454 = Or(x=w1489, y=w1488) -> (x .or. y?=w1445:bool)
            n455 = Or(x=w1445, y=w1446) -> (x .or. y?=w1444:bool)
            n456 = Build Array (concatenate)(w1471, w1452) -> (w1478:dbl[])
            n457 = case shown="True" w1469 {
              tunnel: w1478 -> [_ w1534]
              tunnel: w1476 -> [_ w1536]
              tunnel: w1475 -> [w1533 w1537]
              tunnel: w1474 -> [w1532 w1535]
              tunnel: [w1533 w1539] -> w1473
              tunnel: [w1532 w1538] -> w1472
              frame False {
              }
              frame True {
                n458 = Build Array (concatenate)(w1537, w1536) -> (w1539:dbl[][])
                n459 = Build Array (concatenate)(w1535, w1534) -> (w1538:dbl[][])
              }
            }
            n460 = Reciprocal(x="Sampling Rate (Hz)") -> (1/x=w1482:dbl)
            n461 = Multiply(x=1000.0, y=w1482) -> (x*y=w1480:dbl)
            n462 = case shown="True" w1444 {
              tunnel: w1487 -> [w1574 w1579]
              tunnel: w1486 -> [w1573 w1578]
              tunnel: [w1574 w1576] -> _
              tunnel: [w1573 w1575] -> _
              frame False {
              }
              frame True {
                n463 = call <instrlib>:"Stop.vi"("error in (no error)"=w1579, "Device and Axis"="01", "VISA resource name"=w1578) -> ("error out"=w1576:errorcluster, "VISA resource name out"=w1575:refnum<visa-resource-name>)  [unwired: 7 in]
              }
            }
            n464 = Wait (ms)(milliseconds to wait=w1480) -> ()  [unwired: 1 out]
          }
          n465 = call "Set Speed and Acceleration.vi"("Units (0: data)"=w1284, "New Speed (0)"=w1273, "error in (no error)"=w1287, "Device and Axis"=w1283, "Microstep Size (0)"=w1282, "VISA resource name"=w1288) -> ("error out"=w1286:errorcluster, "VISA resource name out"=w1285:refnum<visa-resource-name>)  [unwired: 4 in]
          n466 = Build Array (concatenate)(w1257, w1266) -> (w1264:dbl[][])
          n467 = Build Array (concatenate)(w1258, w1267) -> (w1265:dbl[][])
          n468 = Negate(x=w1272) -> (-x=w1271:dbl)
          n469 = call "Move.vi"("Units (0: microsteps)"=w1303, "Movement Type (0: relative)"=w1302, "Move Distance (0)"=w1271, "error in (no error)"=w1286, "Device and Axis"=w1283, "Microstep Size (0)"=w1282, "VISA resource name"=w1285) -> ("error out"=w1300:errorcluster, "VISA resource name out"=w1301:refnum<visa-resource-name>)  [unwired: 3 in]
          n470 = while {
            tunnel: w1301 -> [w1378]
            tunnel: w1300 -> [w1377]
            tunnel: [w1350] -> w1299
            tunnel: [w1349] -> w1298
            tunnel: w1280 -> [w1321]
            shift-right: [w1367] -> w1277
            shift-left: w1278 -> [w1368]
            tunnel: w1275 -> [w1363]
            tunnel: w1274 -> [w1348]
            shift-right: [w1335] -> w1260
            shift-left: dbl[][] [] ("Array") -> [w1340]
            shift-right: [w1334] -> w1259
            shift-left: dbl[][] [] ("Array") -> [w1339]
            tunnel: w1261 -> [w1341]
            tunnel: w1251 -> [w1333]
            tunnel: w1250 -> [w1329]
            stop <- w1370 stop-if-true
            w1376 = u16 4 items=["microsteps", "microns", "millimeters", "inches", "degrees"] ("Units (0: microsteps)")
            # "in-oz"
            # "Grams"
            n471 = Tick Count (ms)() -> (millisecond timer value=w1367:u32)
            n472 = call <vilib>:"High Resolution Relative Seconds.vi"() -> ("relative seconds"=w1332:dbl)
            n473 = Unbundle(w1329) -> (w1328:i32, w1327:i32, w1326:i32, w1325:i32, "new reference"=w1323:refnum<k24>, "DeviceHandle"=w1322:string, w1324:dbl)
            n474 = Unbundle(w1363) -> (w1362:i32, w1361:i32, w1360:i32, w1359:i32, "new reference"=w1358:refnum<k24>, "DeviceHandle"=w1357:string, w1356:dbl)
            n475 = Subtract(x=w1332, y=w1333) -> (x-y=w1331:dbl)
            n476 = Subtract(x=w1367, y=w1368) -> (x-y=w1365:u32)
            n477 = while {
              tunnel: w1358 -> [w1417]
              tunnel: w1357 -> [w1416]
              tunnel: [w1415] -> _
              tunnel: [w1414] -> w1355
              tunnel: [w1413] -> _
              tunnel: [w1411] -> _
              tunnel: [w1410] -> _
              tunnel: w1323 -> [w1406]
              tunnel: w1322 -> [w1405]
              stop <- w1407 continue-if-true
              n478 = invoke class="USB_DLL" method="Normal_Data_Request"(reference=w1417, "DeviceHandle"=w1416) -> (reference out=w1415:refnum<k24>, "Normal_Data_Request"=w1413:string)  [unwired: 3 in, 3 out]
              n479 = invoke class="USB_DLL" method="Normal_Data_Request"(reference=w1406, "DeviceHandle"=w1405) -> ("Normal_Data_Request"=w1411:string)  [unwired: 3 in, 4 out]
              n480 = Equal?(x=w1413, y="Error") -> (x = y?=w1409:bool)
              n481 = Equal?(x=w1411, y="Error") -> (x = y?=w1408:bool)
              n482 = Or(x=w1409, y=w1408) -> (x .or. y?=w1407:bool)
              n483 = Decimal String To Number(string=w1413) -> (number=w1414:i32)  [unwired: 2 in, 1 out]
              n484 = Decimal String To Number(string=w1411) -> (number=w1410:i32)  [unwired: 2 in, 1 out]
            }
            n485 = Divide(x=w1365, y=1000) -> (x/y=w1364:dbl)
            n486 = xnode "Formula"("Get_Offset_Value"=w1362, "Get_Offset_Load"=w1361, "Get_Fullscale_Value"=w1360, "Get_Fullscale_Load"=w1359, "Get_Decimal_Point"=w1356, "Normal_Data_Request"=w1355) -> ("Result"=w1346:dbl)  [unwired: 1 in, 1 out]
            n487 = Reciprocal(x=w1364) -> (1/x=w1338:dbl)
            n488 = xnode "Formula"("Get_Offset_Value"=w1328, "Get_Offset_Load"=w1327, "Get_Fullscale_Value"=w1326, "Get_Fullscale_Load"=w1325, "Get_Decimal_Point"=w1324) -> ("Result"=w1314:dbl)  [unwired: 2 in, 1 out]
            n489 = call "Read Current Position.vi"("Units (0: microsteps)"=w1376, "error in (no error)"=w1377, "Device and Axis"="01", "Microstep Size (0)"=0.000234375, "VISA resource name"=w1378) -> ("error out"=w1372:errorcluster, "Position"=w1373:dbl, "VISA resource name out"=w1371:refnum<visa-resource-name>)  [unwired: 4 in]
            n490 = Build Array(w1373) -> (w1330:dbl[])
            n491 = Greater?(x=w1314, y=800.0) -> (0:w1316:bool)
            n492 = Less?(x=w1314, y=-800.0) -> (x < y?=w1315:bool)
            n493 = local write "1/x"(w1338) -> ()
            n494 = local write "Angle/Time"(w1330) -> ()
            n495 = Subtract(x=w1314, y=w1321) -> (x-y=w1320:dbl)
            n496 = Build Array (concatenate)(w1331, w1330) -> (w1337:dbl[])
            n497 = call "Check for Idle.vi"("error in (no error)"=w1372, "Device and Axis"="00", "VISA resource name"=w1371) -> ("error out"=w1350:errorcluster, "Idle"=w1370:bool, "VISA resource name out"=w1349:refnum<visa-resource-name>)  [unwired: 6 in]
            n498 = Or(x=w1316, y=w1315) -> (x .or. y?=w1312:bool)
            n499 = Subtract(x=w1346, y=w1348) -> (x-y=w1347:dbl)
            n500 = Greater?(x=w1346, y=11.2) -> (0:w1352:bool)
            n501 = Less?(x=w1346, y=-11.2) -> (x < y?=w1351:bool)
            n502 = Build Array(w1320) -> (w1319:dbl[])
            n503 = Or(x=w1352, y=w1351) -> (x .or. y?=w1313:bool)
            n504 = local read "Sampling Rate (Hz)"() -> (w1345:dbl)
            n505 = Build Array(w1347) -> (w1336:dbl[])
            n506 = Build Array (concatenate)(w1336, w1319) -> (w1310:dbl[])
            n507 = case shown="True" w1341 {
              tunnel: w1340 -> [w1398 w1403]
              tunnel: w1339 -> [w1397 w1401]
              tunnel: w1337 -> [_ w1404]
              tunnel: [w1398 w1402] -> w1335
              tunnel: [w1397 w1400] -> w1334
              tunnel: w1310 -> [_ w1399]
              frame False {
              }
              frame True {
                n508 = Build Array (concatenate)(w1403, w1404) -> (w1402:dbl[][])
                n509 = Build Array (concatenate)(w1401, w1399) -> (w1400:dbl[][])
              }
            }
            n510 = Or(x=w1313, y=w1312) -> (x .or. y?=w1311:bool)
            n511 = local write "Torque/Time"(w1336) -> ()
            n512 = local write "Force/Time"(w1319) -> ()
            n513 = case shown="True" w1311 {
              tunnel: w1350 -> [w1438 w1443]
              tunnel: w1349 -> [w1437 w1442]
              tunnel: [w1438 w1440] -> _
              tunnel: [w1437 w1439] -> _
              frame False {
              }
              frame True {
                n514 = call <instrlib>:"Stop.vi"("error in (no error)"=w1443, "Device and Axis"="01", "VISA resource name"=w1442) -> ("error out"=w1440:errorcluster, "VISA resource name out"=w1439:refnum<visa-resource-name>)  [unwired: 7 in]
              }
            }
            n515 = Reciprocal(x=w1345) -> (1/x=w1343:dbl)
            n516 = Multiply(x=1000.0, y=w1343) -> (x*y=w1342:dbl)
            n517 = Wait (ms)(milliseconds to wait=w1342) -> ()  [unwired: 1 out]
          }
          n518 = Build Array (concatenate)(w1256, w1260) -> (w1254:dbl[][])
          n519 = Build Array (concatenate)(w1255, w1259) -> (w1253:dbl[][])
        }
        n520 = Transpose 2D Array(2D array=w1204) -> (transposed array=w1219:dbl[][])
        n521 = Transpose 2D Array(2D array=w1205) -> (transposed array=w1220:dbl[][])
        n522 = Transpose 2D Array(2D array=w1207) -> (transposed array=w1223:dbl[][])
        n523 = Transpose 2D Array(2D array=w1206) -> (transposed array=w1222:dbl[][])
        n524 = Build Array (concatenate)(w1219, w1220) -> (w1221:dbl[][])
        n525 = Transpose 2D Array(2D array=w1221) -> (transposed array=w1225:dbl[][])
        n526 = Build Array (concatenate)(w1222, w1223) -> (w1224:dbl[][])
        n527 = local write "Record Data"(w1215) -> ()
        n528 = Build Array("Time (s)", "Angle (Degrees)", "Torque (in-oz)", "Force (grams)") -> (w1229:string[])
        n529 = Transpose 2D Array(2D array=w1224) -> (transposed array=w1226:dbl[][])
        n530 = local write "On/Off"(w1203) -> ()
        n531 = Build Array (concatenate)(w1225, w1226) -> (w1227:dbl[][])
        n532 = local write "Record Data"(w1203) -> ()
        n533 = call "Sort 2D Array.vim"("index"=0, "2D array"=w1227) -> ("sorted 2D array"=w1228:dbl[][])  [unwired: 8 in, 1 out]
        n534 = Concatenate Strings("Sample Name", ".csv" ("string")) -> (w1217:string)
        n535 = Build Path(base path="Save Folder Path", name or relative path=w1217) -> (appended path=w1230:path)
        n536 = call-poly <vilib>:"Write Delimited Spreadsheet.vi"("file path (dialog if empty)"=w1230, "format (%s)"="%s", "1D data"=w1229, "append to file? (new file:F)"=w1215, "transpose? (no:F)"=FALSE, "delimiter (\\t)"=",") -> ()  [unwired: 8 in, 2 out]
        n537 = call-poly <vilib>:"Write Delimited Spreadsheet.vi"("file path (dialog if empty)"=w1230, "format (%.3f)"="%12.6f", "2D data"=w1228, "append to file? (new file:F)"=w1203, "transpose? (no:F)"=FALSE ("append to file? (new file:F)"), "delimiter (\\t)"=",") -> ()  [unwired: 8 in, 2 out]
      }
      event "CW Button": Value Change {
        w1594 = u16 0 items=["relative", "absolute"] ("Movement Type (0: relative)")
        n538 = event-data() -> ()  [unwired: 1 in, 6 out]
        n539 = call "Move.vi"("Units (0: microsteps)"=w1595, "Movement Type (0: relative)"=w1594, "Move Distance (0)"=w1597, "error in (no error)"=w1592, "Device and Axis"="01", "Microstep Size (0)"=w1596, "VISA resource name"=w1593) -> ("error out"=w1583:errorcluster, "VISA resource name out"=w1582:refnum<visa-resource-name>)  [unwired: 3 in]
        n540 = while {
          tunnel: w1584 -> [w1604]
          tunnel: w1583 -> [w1600]
          tunnel: w1582 -> [w1602]
          tunnel: [w1603] -> w1581
          tunnel: [w1599] -> w1580
          stop <- w1601 stop-if-true
          n541 = Unbundle(w1604) -> (w1613:i32, w1612:i32, w1611:i32, w1610:i32, "new reference"=w1608:refnum<k24>, "DeviceHandle"=w1609:string, w1607:dbl)
          n542 = while {
            tunnel: [w1630] -> w1618
            tunnel: w1608 -> [w1629]
            tunnel: [w1628] -> _
            tunnel: w1609 -> [w1627]
            tunnel: [w1626] -> _
            stop <- w1631 continue-if-true
            n543 = invoke class="USB_DLL" method="Normal_Data_Request"(reference=w1629, "DeviceHandle"=w1627) -> (reference out=w1628:refnum<k24>, "Normal_Data_Request"=w1626:string)  [unwired: 3 in, 3 out]
            n544 = Equal?(x=w1626, y="Error") -> (x = y?=w1631:bool)
            n545 = Decimal String To Number(string=w1626) -> (number=w1630:i32)  [unwired: 2 in, 1 out]
          }
          n546 = xnode "Formula"("Get_Offset_Value"=w1613, "Get_Offset_Load"=w1612, "Get_Fullscale_Value"=w1611, "Get_Fullscale_Load"=w1610, "Get_Decimal_Point"=w1607, "Normal_Data_Request"=w1618) -> ("Result"=w1606:dbl)  [unwired: 1 in, 1 out]
          n547 = Build Array(w1606) -> (w1605:dbl[])
          n548 = local write "Torque/Time"(w1605) -> ()
          n549 = Less?(x=w1606, y=-11.2) -> (x < y?=w1616:bool)
          n550 = Greater?(x=w1606, y=11.2) -> (0:w1617:bool)
          n551 = Or(x=w1617, y=w1616) -> (x .or. y?=w1598:bool)
          n552 = case shown="True" w1598 {
            tunnel: w1602 -> [w1620 w1625]
            tunnel: w1600 -> [w1619 w1624]
            tunnel: [w1620 w1622] -> _
            tunnel: [w1619 w1621] -> _
            frame False {
            }
            frame True {
              n553 = call <instrlib>:"Stop.vi"("error in (no error)"=w1624, "Device and Axis"="01", "VISA resource name"=w1625) -> ("error out"=w1621:errorcluster, "VISA resource name out"=w1622:refnum<visa-resource-name>)  [unwired: 7 in]
            }
          }
          n554 = call "Check for Idle.vi"("error in (no error)"=w1600, "VISA resource name"=w1602) -> ("error out"=w1599:errorcluster, "Idle"=w1601:bool, "VISA resource name out"=w1603:refnum<visa-resource-name>)  [unwired: 7 in]
        }
      }
      event "CCW Button": Value Change {
        w1664 = u16 0 items=["relative", "absolute"] ("Movement Type (0: relative)")
        n555 = event-data() -> ()  [unwired: 1 in, 6 out]
        n556 = Negate(x=w1670) -> (-x=w1669:dbl)
        n557 = call "Move.vi"("Units (0: microsteps)"=w1668, "Movement Type (0: relative)"=w1664, "Move Distance (0)"=w1669, "error in (no error)"=w1665, "Device and Axis"="01", "Microstep Size (0)"=w1667, "VISA resource name"=w1666) -> ("error out"=w1653:errorcluster, "VISA resource name out"=w1654:refnum<visa-resource-name>)  [unwired: 3 in]
        n558 = while {
          tunnel: w1655 -> [w1677]
          tunnel: w1653 -> [w1673]
          tunnel: w1654 -> [w1675]
          tunnel: [w1676] -> w1652
          tunnel: [w1672] -> w1651
          stop <- w1674 stop-if-true
          n559 = Unbundle(w1677) -> (w1686:i32, w1685:i32, w1684:i32, w1683:i32, "new reference"=w1681:refnum<k24>, "DeviceHandle"=w1682:string, w1680:dbl)
          n560 = while {
            tunnel: [w1703] -> w1691
            tunnel: w1681 -> [w1702]
            tunnel: [w1701] -> _
            tunnel: w1682 -> [w1700]
            tunnel: [w1699] -> _
            stop <- w1704 continue-if-true
            n561 = invoke class="USB_DLL" method="Normal_Data_Request"(reference=w1702, "DeviceHandle"=w1700) -> (reference out=w1701:refnum<k24>, "Normal_Data_Request"=w1699:string)  [unwired: 3 in, 3 out]
            n562 = Equal?(x=w1699, y="Error") -> (x = y?=w1704:bool)
            n563 = Decimal String To Number(string=w1699) -> (number=w1703:i32)  [unwired: 2 in, 1 out]
          }
          n564 = xnode "Formula"("Get_Offset_Value"=w1686, "Get_Offset_Load"=w1685, "Get_Fullscale_Value"=w1684, "Get_Fullscale_Load"=w1683, "Get_Decimal_Point"=w1680, "Normal_Data_Request"=w1691) -> ("Result"=w1679:dbl)  [unwired: 1 in, 1 out]
          n565 = Build Array(w1679) -> (w1678:dbl[])
          n566 = local write "Torque/Time"(w1678) -> ()
          n567 = Less?(x=w1679, y=-11.2) -> (x < y?=w1689:bool)
          n568 = Greater?(x=w1679, y=11.2) -> (0:w1690:bool)
          n569 = Or(x=w1690, y=w1689) -> (x .or. y?=w1671:bool)
          n570 = case shown="True" w1671 {
            tunnel: w1675 -> [w1693 w1698]
            tunnel: w1673 -> [w1692 w1697]
            tunnel: [w1693 w1695] -> _
            tunnel: [w1692 w1694] -> _
            frame False {
            }
            frame True {
              n571 = call <instrlib>:"Stop.vi"("error in (no error)"=w1697, "Device and Axis"="01", "VISA resource name"=w1698) -> ("error out"=w1694:errorcluster, "VISA resource name out"=w1695:refnum<visa-resource-name>)  [unwired: 7 in]
            }
          }
          n572 = call "Check for Idle.vi"("error in (no error)"=w1673, "VISA resource name"=w1675) -> ("error out"=w1672:errorcluster, "Idle"=w1674:bool, "VISA resource name out"=w1676:refnum<visa-resource-name>)  [unwired: 7 in]
        }
      }
      event "Home Button": Value Change {
        n573 = event-data() -> ()  [unwired: 1 in, 6 out]
        n574 = call "Prompt User for Input"() -> ("OK"=w1726:bool)  [unwired: 18 in, 1 out]
        n575 = case shown="True" w1726 {
          tunnel: w1728 -> [w1736 w1742]
          tunnel: w1727 -> [w1737 w1740]
          tunnel: [w1737 w1739] -> w1725
          tunnel: [w1736 w1738] -> w1724
          frame False {
          }
          frame True {
            n576 = call "Home.vi"("error in (no error)"=w1742, "Device and Axis"="00", "VISA resource name"=w1740) -> ("error out"=w1738:errorcluster, "VISA resource name out"=w1739:refnum<visa-resource-name>)  [unwired: 7 in]
          }
        }
      }
      event "Save Button": Value Change {
        n577 = event-data() -> ()  [unwired: 1 in, 6 out]
        n578 = call "Read Current Position.vi"("Units (0: microsteps)"=w1753, "error in (no error)"=w1751, "Device and Axis"="01", "Microstep Size (0)"=w1754, "VISA resource name"=w1752) -> ("error out"=w1748:errorcluster, "Position"=w1744:dbl, "VISA resource name out"=w1749:refnum<visa-resource-name>)  [unwired: 4 in]
        n579 = Negate(x=w1744) -> (-x=w1743:dbl)
        n580 = Build Array(w1743) -> (w1745:dbl[])
      }
    }
    n581 = Bundle("new reference"=w172, "DeviceHandle"=w171) -> (w170:T3)  [unwired: 1 in]
    n582 = Bundle("new reference"=w153, "DeviceHandle"=w152) -> (w151:T3)  [unwired: 1 in]
    n583 = local write "On/Off"(TRUE) -> ()
    n584 = Unbundle(w170) -> ("new reference"=w169:refnum<k24>, "DeviceHandle"=w168:string)
    n585 = Unbundle(w151) -> ("new reference"=w150:refnum<k24>, "DeviceHandle"=w149:string)
  }
  n586 = flat-sequence {
    tunnel: w20 -> [w1767]
    tunnel: w15 -> [w1764]
    tunnel: w14 -> [w1763]
    tunnel: w13 -> [w1762]
    tunnel: w8 -> [w1761]
    tunnel: w1 -> [w1757]
    tunnel: w5 -> [w1756]
    tunnel: w3 -> [w1759]
    tunnel: w2 -> [w1758]
    frame #0 {
      n587 = invoke class="MG17Motor" method="StopCtrl"(reference=w1757, error in=w1756) -> (error out=→"error out":errorcluster)  [unwired: 1 in, 2 out]
      n588 = call "Close.vi"("error in (no error)"=w1762, "VISA resource name"=w1767) -> ("error out"=w1766:errorcluster)  [unwired: 9 in]
      n589 = invoke class="USB_DLL" method="Close_Device_Connection"(reference=w1759, "DeviceHandle"=w1758) -> (reference out=w1760:refnum<k24>)  [unwired: 2 in, 3 out]
      n590 = invoke class="USB_DLL" method="Close_Device_Connection"(reference=w1764, "DeviceHandle"=w1763) -> (reference out=w1765:refnum<k24>)  [unwired: 2 in, 3 out]
      n591 = call <vilib>:"Simple Error Handler.vi"("error in (no error)"=w1766) -> ()  [unwired: 4 in, 5 out]
      n592 = Close Reference(reference=w1760) -> ()  [unwired: 1 in, 1 out]
      n593 = Close Reference(reference=w1765) -> ()  [unwired: 1 in, 1 out]
      "Saved Position" <- w1761
    }
  }
